vi "01 Washer HCC.vi"() -> ()   [LabVIEW 2009]
uses:
  Washer.ctl
  Dryer Wilt/Dryer Details.ctl
  Dryer Wilt/Dryer.ctl
  Dryer Wilt/Agilent Channel Definition.ctl
  Dryer Wilt/Dryer Com Port Info.ctl
  Dryer Wilt/Dryer Status Ctrl.ctl
  Dryer Wilt/Dryer Test State.ctl
  <vilib>/Platform/fileVersionInfo.llb/FileVersionInformation.ctl
  Globals HCC.vi
  Dryer Wilt/Update Wilt GUI Control.ctl
  Dryer Wilt/GEA2 Driver/GEA2 Dryer Interface Ctrl.ctl
panel:
  out "User Message":string
  in  "Reset Faults":bool
  in  "Save Setup":bool
  out "Agilent":T1
  out "File Version Info":string
  in  "Robocopy":bool
  out "4":T1
  out "3":T1
  out "2":T1
  out "1A":T1
  out "1":T1
  out "GUI Update":bool=TRUE
  out "Gathering Data Latch":bool=TRUE
  out "Init Complete":bool=TRUE
  out "Dryer Com Info":T2[](array[typedef])=[{"Color"=0, "Last Read Status"=enum."Cycle Not Started", "Command:Data"="", "Com Port"=0, "Time(S)"=0.0, "Err Count"=0}, {"Color"=0, "Last Read Status"=enum."Cycle Not Started", "Command:Data"="", "Com Port"=0, "Time(S)"=0.0, "Err Count"=0}, {"Color"=0, "Last Read Status"=enum."Cycle Not Started", "Command:Data"="", "Com Port"=0, "Time(S)"=0.0, "Err Count"=0}, {"Color"=0, "Last Read Status"=enum."Cycle Not Started", "Command:Data"="", "Com Port"=0, "Time(S)"=0.0, "Err Count"=0}, {"Color"=0, "Last Read Status"=enum."Cycle Not Started", "Command:Data"="", "Com Port"=0, "Time(S)"=0.0, "Err Count"=0}, {"Color"=0, "Last Read Status"=enum."Cycle Not Started", "Command:Data"="", "Com Port"=0, "Time(S)"=0.0, "Err Count"=0}, {"Color"=0, "Last Read Status"=enum."Cycle Not Started", "Command:Data"="", "Com Port"=0, "Time(S)"=0.0, "Err Count"=0}, {"Color"=0, "Last Read Status"=enum."Cycle Not Started", "Command:Data"="", "Com Port"=0, "Time(S)"=0.0, "Err Count"=0}, {"Color"=0, "Last Read Status"=enum."Cycle Not Started", "Command:Data"="", "Com Port"=0, "Time(S)"=0.0, "Err Count"=0}, {"Color"=0, "Last Read Status"=enum."Cycle Not Started", "Command:Data"="", "Com Port"=0, "Time(S)"=0.0, "Err Count"=0}, {"Color"=0, "Last Read Status"=enum."Cycle Not Started", "Command:Data"="", "Com Port"=0, "Time(S)"=0.0, "Err Count"=0}, {"Color"=0, "Last Read Status"=enum."Cycle Not Started", "Command:Data"="", "Com Port"=0, "Time(S)"=0.0, "Err Count"=0}, {"Color"=0, "Last Read Status"=enum."Cycle Not Started", "Command:Data"="", "Com Port"=0, "Time(S)"=0.0, "Err Count"=0}, {"Color"=0, "Last Read Status"=enum."Cycle Not Started", "Command:Data"="", "Com Port"=0, "Time(S)"=0.0, "Err Count"=0}, {"Color"=0, "Last Read Status"=enum."Cycle Not Started", "Command:Data"="", "Com Port"=0, "Time(S)"=0.0, "Err Count"=0}, {"Color"=0, "Last Read Status"=enum."Cycle Not Started", "Command:Data"="", "Com Port"=0, "Time(S)"=0.0, "Err Count"=0}, {"Color"=0, "Last Read Status"=enum."Cycle Not Started", "Command:Data"="", "Com Port"=0, "Time(S)"=0.0, "Err Count"=0}, {"Color"=0, "Last Read Status"=enum."Cycle Not Started", "Command:Data"="", "Com Port"=0, "Time(S)"=0.0, "Err Count"=0}, {"Color"=0, "Last Read Status"=enum."Cycle Not Started", "Command:Data"="", "Com Port"=0, "Time(S)"=0.0, "Err Count"=0}, {"Color"=0, "Last Read Status"=enum."Cycle Not Started", "Command:Data"="", "Com Port"=0, "Time(S)"=0.0, "Err Count"=0}, {"Color"=0, "Last Read Status"=enum."Cycle Not Started", "Command:Data"="", "Com Port"=0, "Time(S)"=0.0, "Err Count"=0}, {"Color"=0, "Last Read Status"=enum."Cycle Not Started", "Command:Data"="", "Com Port"=0, "Time(S)"=0.0, "Err Count"=0}, {"Color"=0, "Last Read Status"=enum."Cycle Not Started", "Command:Data"="", "Com Port"=0, "Time(S)"=0.0, "Err Count"=0}, {"Color"=0, "Last Read Status"=enum."Cycle Not Started", "Command:Data"="", "Com Port"=0, "Time(S)"=0.0, "Err Count"=0}, {"Color"=0, "Last Read Status"=enum."Cycle Not Started", "Command:Data"="", "Com Port"=0, "Time(S)"=0.0, "Err Count"=0}, {"Color"=0, "Last Read Status"=enum."Cycle Not Started", "Command:Data"="", "Com Port"=0, "Time(S)"=0.0, "Err Count"=0}, {"Color"=0, "Last Read Status"=enum."Cycle Not Started", "Command:Data"="", "Com Port"=0, "Time(S)"=0.0, "Err Count"=0}, {"Color"=0, "Last Read Status"=enum."Cycle Not Started", "Command:Data"="", "Com Port"=0, "Time(S)"=0.0, "Err Count"=0}, {"Color"=0, "Last Read Status"=enum."Cycle Not Started", "Command:Data"="", "Com Port"=0, "Time(S)"=0.0, "Err Count"=0}, {"Color"=0, "Last Read Status"=enum."Cycle Not Started", "Command:Data"="", "Com Port"=0, "Time(S)"=0.0, "Err Count"=0}, {"Color"=0, "Last Read Status"=enum."Cycle Not Started", "Command:Data"="", "Com Port"=0, "Time(S)"=0.0, "Err Count"=0}, {"Color"=0, "Last Read Status"=enum."Cycle Not Started", "Command:Data"="", "Com Port"=0, "Time(S)"=0.0, "Err Count"=0}, {"Color"=0, "Last Read Status"=enum."Cycle Not Started", "Command:Data"="", "Com Port"=0, "Time(S)"=0.0, "Err Count"=0}, {"Color"=0, "Last Read Status"=enum."Cycle Not Started", "Command:Data"="", "Com Port"=0, "Time(S)"=0.0, "Err Count"=0}, {"Color"=0, "Last Read Status"=enum."Cycle Not Started", "Command:Data"="", "Com Port"=0, "Time(S)"=0.0, "Err Count"=0}, {"Color"=0, "Last Read Status"=enum."Cycle Not Started", "Command:Data"="", "Com Port"=0, "Time(S)"=0.0, "Err Count"=0}, {"Color"=0, "Last Read Status"=enum."Cycle Not Started", "Command:Data"="", "Com Port"=0, "Time(S)"=0.0, "Err Count"=0}, {"Color"=0, "Last Read Status"=enum."Cycle Not Started", "Command:Data"="", "Com Port"=0, "Time(S)"=0.0, "Err Count"=0}, {"Color"=0, "Last Read Status"=enum."Cycle Not Started", "Command:Data"="", "Com Port"=0, "Time(S)"=0.0, "Err Count"=0}, {"Color"=0, "Last Read Status"=enum."Cycle Not Started", "Command:Data"="", "Com Port"=0, "Time(S)"=0.0, "Err Count"=0}, {"Color"=0, "Last Read Status"=enum."Cycle Not Started", "Command:Data"="", "Com Port"=0, "Time(S)"=0.0, "Err Count"=0}, {"Color"=0, "Last Read Status"=enum."Cycle Not Started", "Command:Data"="", "Com Port"=0, "Time(S)"=0.0, "Err Count"=0}, {"Color"=0, "Last Read Status"=enum."Cycle Not Started", "Command:Data"="", "Com Port"=0, "Time(S)"=0.0, "Err Count"=0}, {"Color"=0, "Last Read Status"=enum."Cycle Not Started", "Command:Data"="", "Com Port"=0, "Time(S)"=0.0, "Err Count"=0}, {"Color"=0, "Last Read Status"=enum."Cycle Not Started", "Command:Data"="", "Com Port"=0, "Time(S)"=0.0, "Err Count"=0}, {"Color"=0, "Last Read Status"=enum."Cycle Not Started", "Command:Data"="", "Com Port"=0, "Time(S)"=0.0, "Err Count"=0}, {"Color"=0, "Last Read Status"=enum."Cycle Not Started", "Command:Data"="", "Com Port"=0, "Time(S)"=0.0, "Err Count"=0}, {"Color"=0, "Last Read Status"=enum."Cycle Not Started", "Command:Data"="", "Com Port"=0, "Time(S)"=0.0, "Err Count"=0}, {"Color"=0, "Last Read Status"=enum."Cycle Not Started", "Command:Data"="", "Com Port"=0, "Time(S)"=0.0, "Err Count"=0}, {"Color"=0, "Last Read Status"=enum."Cycle Not Started", "Command:Data"="", "Com Port"=0, "Time(S)"=0.0, "Err Count"=0}, {"Color"=0, "Last Read Status"=enum."Cycle Not Started", "Command:Data"="", "Com Port"=0, "Time(S)"=0.0, "Err Count"=0}, {"Color"=0, "Last Read Status"=enum."Cycle Not Started", "Command:Data"="", "Com Port"=0, "Time(S)"=0.0, "Err Count"=0}, {"Color"=0, "Last Read Status"=enum."Cycle Not Started", "Command:Data"="", "Com Port"=0, "Time(S)"=0.0, "Err Count"=0}, {"Color"=0, "Last Read Status"=enum."Cycle Not Started", "Command:Data"="", "Com Port"=0, "Time(S)"=0.0, "Err Count"=0}, {"Color"=0, "Last Read Status"=enum."Cycle Not Started", "Command:Data"="", "Com Port"=0, "Time(S)"=0.0, "Err Count"=0}, {"Color"=0, "Last Read Status"=enum."Cycle Not Started", "Command:Data"="", "Com Port"=0, "Time(S)"=0.0, "Err Count"=0}, {"Color"=0, "Last Read Status"=enum."Cycle Not Started", "Command:Data"="", "Com Port"=0, "Time(S)"=0.0, "Err Count"=0}, {"Color"=0, "Last Read Status"=enum."Cycle Not Started", "Command:Data"="", "Com Port"=0, "Time(S)"=0.0, "Err Count"=0}, {"Color"=0, "Last Read Status"=enum."Cycle Not Started", "Command:Data"="", "Com Port"=0, "Time(S)"=0.0, "Err Count"=0}, {"Color"=0, "Last Read Status"=enum."Cycle Not Started", "Command:Data"="", "Com Port"=0, "Time(S)"=0.0, "Err Count"=0}, {"Color"=0, "Last Read Status"=enum."Cycle Not Started", "Command:Data"="", "Com Port"=0, "Time(S)"=0.0, "Err Count"=0}, {"Color"=0, "Last Read Status"=enum."Cycle Not Started", "Command:Data"="", "Com Port"=0, "Time(S)"=0.0, "Err Count"=0}, {"Color"=0, "Last Read Status"=enum."Cycle Not Started", "Command:Data"="", "Com Port"=0, "Time(S)"=0.0, "Err Count"=0}, {"Color"=0, "Last Read Status"=enum."Cycle Not Started", "Command:Data"="", "Com Port"=0, "Time(S)"=0.0, "Err Count"=0}, {"Color"=0, "Last Read Status"=enum."Cycle Not Started", "Command:Data"="", "Com Port"=0, "Time(S)"=0.0, "Err Count"=0}, {"Color"=0, "Last Read Status"=enum."Cycle Not Started", "Command:Data"="", "Com Port"=0, "Time(S)"=0.0, "Err Count"=0}, {"Color"=0, "Last Read Status"=enum."Cycle Not Started", "Command:Data"="", "Com Port"=0, "Time(S)"=0.0, "Err Count"=0}, {"Color"=0, "Last Read Status"=enum."Cycle Not Started", "Command:Data"="", "Com Port"=0, "Time(S)"=0.0, "Err Count"=0}, {"Color"=0, "Last Read Status"=enum."Cycle Not Started", "Command:Data"="", "Com Port"=0, "Time(S)"=0.0, "Err Count"=0}, {"Color"=0, "Last Read Status"=enum."Cycle Not Started", "Command:Data"="", "Com Port"=0, "Time(S)"=0.0, "Err Count"=0}, {"Color"=0, "Last Read Status"=enum."Cycle Not Started", "Command:Data"="", "Com Port"=0, "Time(S)"=0.0, "Err Count"=0}, {"Color"=0, "Last Read Status"=enum."Cycle Not Started", "Command:Data"="", "Com Port"=0, "Time(S)"=0.0, "Err Count"=0}, {"Color"=0, "Last Read Status"=enum."Cycle Not Started", "Command:Data"="", "Com Port"=0, "Time(S)"=0.0, "Err Count"=0}, {"Color"=0, "Last Read Status"=enum."Cycle Not Started", "Command:Data"="", "Com Port"=0, "Time(S)"=0.0, "Err Count"=0}, {"Color"=0, "Last Read Status"=enum."Cycle Not Started", "Command:Data"="", "Com Port"=0, "Time(S)"=0.0, "Err Count"=0}, {"Color"=0, "Last Read Status"=enum."Cycle Not Started", "Command:Data"="", "Com Port"=0, "Time(S)"=0.0, "Err Count"=0}, {"Color"=0, "Last Read Status"=enum."Cycle Not Started", "Command:Data"="", "Com Port"=0, "Time(S)"=0.0, "Err Count"=0}, {"Color"=0, "Last Read Status"=enum."Cycle Not Started", "Command:Data"="", "Com Port"=0, "Time(S)"=0.0, "Err Count"=0}, {"Color"=0, "Last Read Status"=enum."Cycle Not Started", "Command:Data"="", "Com Port"=0, "Time(S)"=0.0, "Err Count"=0}, {"Color"=0, "Last Read Status"=enum."Cycle Not Started", "Command:Data"="", "Com Port"=0, "Time(S)"=0.0, "Err Count"=0}, {"Color"=0, "Last Read Status"=enum."Cycle Not Started", "Command:Data"="", "Com Port"=0, "Time(S)"=0.0, "Err Count"=0}, {"Color"=0, "Last Read Status"=enum."Cycle Not Started", "Command:Data"="", "Com Port"=0, "Time(S)"=0.0, "Err Count"=0}, {"Color"=0, "Last Read Status"=enum."Cycle Not Started", "Command:Data"="", "Com Port"=0, "Time(S)"=0.0, "Err Count"=0}, {"Color"=0, "Last Read Status"=enum."Cycle Not Started", "Command:Data"="", "Com Port"=0, "Time(S)"=0.0, "Err Count"=0}, {"Color"=0, "Last Read Status"=enum."Cycle Not Started", "Command:Data"="", "Com Port"=0, "Time(S)"=0.0, "Err Count"=0}, {"Color"=0, "Last Read Status"=enum."Cycle Not Started", "Command:Data"="", "Com Port"=0, "Time(S)"=0.0, "Err Count"=0}, {"Color"=0, "Last Read Status"=enum."Cycle Not Started", "Command:Data"="", "Com Port"=0, "Time(S)"=0.0, "Err Count"=0}, {"Color"=0, "Last Read Status"=enum."Cycle Not Started", "Command:Data"="", "Com Port"=0, "Time(S)"=0.0, "Err Count"=0}, {"Color"=0, "Last Read Status"=enum."Cycle Not Started", "Command:Data"="", "Com Port"=0, "Time(S)"=0.0, "Err Count"=0}, {"Color"=0, "Last Read Status"=enum."Cycle Not Started", "Command:Data"="", "Com Port"=0, "Time(S)"=0.0, "Err Count"=0}, {"Color"=0, "Last Read Status"=enum."Cycle Not Started", "Command:Data"="", "Com Port"=0, "Time(S)"=0.0, "Err Count"=0}, {"Color"=0, "Last Read Status"=enum."Cycle Not Started", "Command:Data"="", "Com Port"=0, "Time(S)"=0.0, "Err Count"=0}, {"Color"=0, "Last Read Status"=enum."Cycle Not Started", "Command:Data"="", "Com Port"=0, "Time(S)"=0.0, "Err Count"=0}, {"Color"=0, "Last Read Status"=enum."Cycle Not Started", "Command:Data"="", "Com Port"=0, "Time(S)"=0.0, "Err Count"=0}, {"Color"=0, "Last Read Status"=enum."Cycle Not Started", "Command:Data"="", "Com Port"=0, "Time(S)"=0.0, "Err Count"=0}, {"Color"=0, "Last Read Status"=enum."Cycle Not Started", "Command:Data"="", "Com Port"=0, "Time(S)"=0.0, "Err Count"=0}, {"Color"=0, "Last Read Status"=enum."Cycle Not Started", "Command:Data"="", "Com Port"=0, "Time(S)"=0.0, "Err Count"=0}, {"Color"=0, "Last Read Status"=enum."Cycle Not Started", "Command:Data"="", "Com Port"=0, "Time(S)"=0.0, "Err Count"=0}, {"Color"=0, "Last Read Status"=enum."Cycle Not Started", "Command:Data"="", "Com Port"=0, "Time(S)"=0.0, "Err Count"=0}, {"Color"=0, "Last Read Status"=enum."Cycle Not Started", "Command:Data"="", "Com Port"=0, "Time(S)"=0.0, "Err Count"=0}, {"Color"=0, "Last Read Status"=enum."Cycle Not Started", "Command:Data"="", "Com Port"=0, "Time(S)"=0.0, "Err Count"=0}, {"Color"=0, "Last Read Status"=enum."Cycle Not Started", "Command:Data"="", "Com Port"=0, "Time(S)"=0.0, "Err Count"=0}, {"Color"=0, "Last Read Status"=enum."Cycle Not Started", "Command:Data"="", "Com Port"=0, "Time(S)"=0.0, "Err Count"=0}, {"Color"=0, "Last Read Status"=enum."Cycle Not Started", "Command:Data"="", "Com Port"=0, "Time(S)"=0.0, "Err Count"=0}, {"Color"=0, "Last Read Status"=enum."Cycle Not Started", "Command:Data"="", "Com Port"=0, "Time(S)"=0.0, "Err Count"=0}, {"Color"=0, "Last Read Status"=enum."Cycle Not Started", "Command:Data"="", "Com Port"=0, "Time(S)"=0.0, "Err Count"=0}, {"Color"=0, "Last Read Status"=enum."Cycle Not Started", "Command:Data"="", "Com Port"=0, "Time(S)"=0.0, "Err Count"=0}, {"Color"=0, "Last Read Status"=enum."Cycle Not Started", "Command:Data"="", "Com Port"=0, "Time(S)"=0.0, "Err Count"=0}, {"Color"=0, "Last Read Status"=enum."Cycle Not Started", "Command:Data"="", "Com Port"=0, "Time(S)"=0.0, "Err Count"=0}, {"Color"=0, "Last Read Status"=enum."Cycle Not Started", "Command:Data"="", "Com Port"=0, "Time(S)"=0.0, "Err Count"=0}, {"Color"=0, "Last Read Status"=enum."Cycle Not Started", "Command:Data"="", "Com Port"=0, "Time(S)"=0.0, "Err Count"=0}, {"Color"=0, "Last Read Status"=enum."Cycle Not Started", "Command:Data"="", "Com Port"=0, "Time(S)"=0.0, "Err Count"=0}, {"Color"=0, "Last Read Status"=enum."Cycle Not Started", "Command:Data"="", "Com Port"=0, "Time(S)"=0.0, "Err Count"=0}, {"Color"=0, "Last Read Status"=enum."Cycle Not Started", "Command:Data"="", "Com Port"=0, "Time(S)"=0.0, "Err Count"=0}, {"Color"=0, "Last Read Status"=enum."Cycle Not Started", "Command:Data"="", "Com Port"=0, "Time(S)"=0.0, "Err Count"=0}, {"Color"=0, "Last Read Status"=enum."Cycle Not Started", "Command:Data"="", "Com Port"=0, "Time(S)"=0.0, "Err Count"=0}, {"Color"=0, "Last Read Status"=enum."Cycle Not Started", "Command:Data"="", "Com Port"=0, "Time(S)"=0.0, "Err Count"=0}, {"Color"=0, "Last Read Status"=enum."Cycle Not Started", "Command:Data"="", "Com Port"=0, "Time(S)"=0.0, "Err Count"=0}, {"Color"=0, "Last Read Status"=enum."Cycle Not Started", "Command:Data"="", "Com Port"=0, "Time(S)"=0.0, "Err Count"=0}, {"Color"=0, "Last Read Status"=enum."Cycle Not Started", "Command:Data"="", "Com Port"=0, "Time(S)"=0.0, "Err Count"=0}, {"Color"=0, "Last Read Status"=enum."Cycle Not Started", "Command:Data"="", "Com Port"=0, "Time(S)"=0.0, "Err Count"=0}, {"Color"=0, "Last Read Status"=enum."Cycle Not Started", "Command:Data"="", "Com Port"=0, "Time(S)"=0.0, "Err Count"=0}, {"Color"=0, "Last Read Status"=enum."Cycle Not Started", "Command:Data"="", "Com Port"=0, "Time(S)"=0.0, "Err Count"=0}, {"Color"=0, "Last Read Status"=enum."Cycle Not Started", "Command:Data"="", "Com Port"=0, "Time(S)"=0.0, "Err Count"=0}, {"Color"=0, "Last Read Status"=enum."Cycle Not Started", "Command:Data"="", "Com Port"=0, "Time(S)"=0.0, "Err Count"=0}, {"Color"=0, "Last Read Status"=enum."Cycle Not Started", "Command:Data"="", "Com Port"=0, "Time(S)"=0.0, "Err Count"=0}, {"Color"=0, "Last Read Status"=enum."Cycle Not Started", "Command:Data"="", "Com Port"=0, "Time(S)"=0.0, "Err Count"=0}, {"Color"=0, "Last Read Status"=enum."Cycle Not Started", "Command:Data"="", "Com Port"=0, "Time(S)"=0.0, "Err Count"=0}, {"Color"=0, "Last Read Status"=enum."Cycle Not Started", "Command:Data"="", "Com Port"=0, "Time(S)"=0.0, "Err Count"=0}, {"Color"=0, "Last Read Status"=enum."Cycle Not Started", "Command:Data"="", "Com Port"=0, "Time(S)"=0.0, "Err Count"=0}, {"Color"=0, "Last Read Status"=enum."Cycle Not Started", "Command:Data"="", "Com Port"=0, "Time(S)"=0.0, "Err Count"=0}, {"Color"=0, "Last Read Status"=enum."Cycle Not Started", "Command:Data"="", "Com Port"=0, "Time(S)"=0.0, "Err Count"=0}, {"Color"=0, "Last Read Status"=enum."Cycle Not Started", "Command:Data"="", "Com Port"=0, "Time(S)"=0.0, "Err Count"=0}, {"Color"=0, "Last Read Status"=enum."Cycle Not Started", "Command:Data"="", "Com Port"=0, "Time(S)"=0.0, "Err Count"=0}, {"Color"=0, "Last Read Status"=enum."Cycle Not Started", "Command:Data"="", "Com Port"=0, "Time(S)"=0.0, "Err Count"=0}, {"Color"=0, "Last Read Status"=enum."Cycle Not Started", "Command:Data"="", "Com Port"=0, "Time(S)"=0.0, "Err Count"=0}, {"Color"=0, "Last Read Status"=enum."Cycle Not Started", "Command:Data"="", "Com Port"=0, "Time(S)"=0.0, "Err Count"=0}, {"Color"=0, "Last Read Status"=enum."Cycle Not Started", "Command:Data"="", "Com Port"=0, "Time(S)"=0.0, "Err Count"=0}, {"Color"=0, "Last Read Status"=enum."Cycle Not Started", "Command:Data"="", "Com Port"=0, "Time(S)"=0.0, "Err Count"=0}, {"Color"=0, "Last Read Status"=enum."Cycle Not Started", "Command:Data"="", "Com Port"=0, "Time(S)"=0.0, "Err Count"=0}, {"Color"=0, "Last Read Status"=enum."Cycle Not Started", "Command:Data"="", "Com Port"=0, "Time(S)"=0.0, "Err Count"=0}, {"Color"=0, "Last Read Status"=enum."Cycle Not Started", "Command:Data"="", "Com Port"=0, "Time(S)"=0.0, "Err Count"=0}, {"Color"=0, "Last Read Status"=enum."Cycle Not Started", "Command:Data"="", "Com Port"=0, "Time(S)"=0.0, "Err Count"=0}, {"Color"=0, "Last Read Status"=enum."Cycle Not Started", "Command:Data"="", "Com Port"=0, "Time(S)"=0.0, "Err Count"=0}, {"Color"=0, "Last Read Status"=enum."Cycle Not Started", "Command:Data"="", "Com Port"=0, "Time(S)"=0.0, "Err Count"=0}, {"Color"=0, "Last Read Status"=enum."Cycle Not Started", "Command:Data"="", "Com Port"=0, "Time(S)"=0.0, "Err Count"=0}, {"Color"=0, "Last Read Status"=enum."Cycle Not Started", "Command:Data"="", "Com Port"=0, "Time(S)"=0.0, "Err Count"=0}, {"Color"=0, "Last Read Status"=enum."Cycle Not Started", "Command:Data"="", "Com Port"=0, "Time(S)"=0.0, "Err Count"=0}, {"Color"=0, "Last Read Status"=enum."Cycle Not Started", "Command:Data"="", "Com Port"=0, "Time(S)"=0.0, "Err Count"=0}, {"Color"=0, "Last Read Status"=enum."Cycle Not Started", "Command:Data"="", "Com Port"=0, "Time(S)"=0.0, "Err Count"=0}, {"Color"=0, "Last Read Status"=enum."Cycle Not Started", "Command:Data"="", "Com Port"=0, "Time(S)"=0.0, "Err Count"=0}, {"Color"=0, "Last Read Status"=enum."Cycle Not Started", "Command:Data"="", "Com Port"=0, "Time(S)"=0.0, "Err Count"=0}, {"Color"=0, "Last Read Status"=enum."Cycle Not Started", "Command:Data"="", "Com Port"=0, "Time(S)"=0.0, "Err Count"=0}, {"Color"=0, "Last Read Status"=enum."Cycle Not Started", "Command:Data"="", "Com Port"=0, "Time(S)"=0.0, "Err Count"=0}, {"Color"=0, "Last Read Status"=enum."Cycle Not Started", "Command:Data"="", "Com Port"=0, "Time(S)"=0.0, "Err Count"=0}, {"Color"=0, "Last Read Status"=enum."Cycle Not Started", "Command:Data"="", "Com Port"=0, "Time(S)"=0.0, "Err Count"=0}, {"Color"=0, "Last Read Status"=enum."Cycle Not Started", "Command:Data"="", "Com Port"=0, "Time(S)"=0.0, "Err Count"=0}, {"Color"=0, "Last Read Status"=enum."Cycle Not Started", "Command:Data"="", "Com Port"=0, "Time(S)"=0.0, "Err Count"=0}, {"Color"=0, "Last Read Status"=enum."Cycle Not Started", "Command:Data"="", "Com Port"=0, "Time(S)"=0.0, "Err Count"=0}, {"Color"=0, "Last Read Status"=enum."Cycle Not Started", "Command:Data"="", "Com Port"=0, "Time(S)"=0.0, "Err Count"=0}, {"Color"=0, "Last Read Status"=enum."Cycle Not Started", "Command:Data"="", "Com Port"=0, "Time(S)"=0.0, "Err Count"=0}, {"Color"=0, "Last Read Status"=enum."Cycle Not Started", "Command:Data"="", "Com Port"=0, "Time(S)"=0.0, "Err Count"=0}, {"Color"=0, "Last Read Status"=enum."Cycle Not Started", "Command:Data"="", "Com Port"=0, "Time(S)"=0.0, "Err Count"=0}, {"Color"=0, "Last Read Status"=enum."Cycle Not Started", "Command:Data"="", "Com Port"=0, "Time(S)"=0.0, "Err Count"=0}, {"Color"=0, "Last Read Status"=enum."Cycle Not Started", "Command:Data"="", "Com Port"=0, "Time(S)"=0.0, "Err Count"=0}, {"Color"=0, "Last Read Status"=enum."Cycle Not Started", "Command:Data"="", "Com Port"=0, "Time(S)"=0.0, "Err Count"=0}, {"Color"=0, "Last Read Status"=enum."Cycle Not Started", "Command:Data"="", "Com Port"=0, "Time(S)"=0.0, "Err Count"=0}, {"Color"=0, "Last Read Status"=enum."Cycle Not Started", "Command:Data"="", "Com Port"=0, "Time(S)"=0.0, "Err Count"=0}, {"Color"=0, "Last Read Status"=enum."Cycle Not Started", "Command:Data"="", "Com Port"=0, "Time(S)"=0.0, "Err Count"=0}, {"Color"=0, "Last Read Status"=enum."Cycle Not Started", "Command:Data"="", "Com Port"=0, "Time(S)"=0.0, "Err Count"=0}, {"Color"=0, "Last Read Status"=enum."Cycle Not Started", "Command:Data"="", "Com Port"=0, "Time(S)"=0.0, "Err Count"=0}, {"Color"=0, "Last Read Status"=enum."Cycle Not Started", "Command:Data"="", "Com Port"=0, "Time(S)"=0.0, "Err Count"=0}, {"Color"=0, "Last Read Status"=enum."Cycle Not Started", "Command:Data"="", "Com Port"=0, "Time(S)"=0.0, "Err Count"=0}, {"Color"=0, "Last Read Status"=enum."Cycle Not Started", "Command:Data"="", "Com Port"=0, "Time(S)"=0.0, "Err Count"=0}, {"Color"=0, "Last Read Status"=enum."Cycle Not Started", "Command:Data"="", "Com Port"=0, "Time(S)"=0.0, "Err Count"=0}, {"Color"=0, "Last Read Status"=enum."Cycle Not Started", "Command:Data"="", "Com Port"=0, "Time(S)"=0.0, "Err Count"=0}, {"Color"=0, "Last Read Status"=enum."Cycle Not Started", "Command:Data"="", "Com Port"=0, "Time(S)"=0.0, "Err Count"=0}, {"Color"=0, "Last Read Status"=enum."Cycle Not Started", "Command:Data"="", "Com Port"=0, "Time(S)"=0.0, "Err Count"=0}, {"Color"=0, "Last Read Status"=enum."Cycle Not Started", "Command:Data"="", "Com Port"=0, "Time(S)"=0.0, "Err Count"=0}, {"Color"=0, "Last Read Status"=enum."Cycle Not Started", "Command:Data"="", "Com Port"=0, "Time(S)"=0.0, "Err Count"=0}, {"Color"=0, "Last Read Status"=enum."Cycle Not Started", "Command:Data"="", "Com Port"=0, "Time(S)"=0.0, "Err Count"=0}, {"Color"=0, "Last Read Status"=enum."Cycle Not Started", "Command:Data"="", "Com Port"=0, "Time(S)"=0.0, "Err Count"=0}, {"Color"=0, "Last Read Status"=enum."Cycle Not Started", "Command:Data"="", "Com Port"=0, "Time(S)"=0.0, "Err Count"=0}, {"Color"=0, "Last Read Status"=enum."Cycle Not Started", "Command:Data"="", "Com Port"=0, "Time(S)"=0.0, "Err Count"=0}, {"Color"=0, "Last Read Status"=enum."Cycle Not Started", "Command:Data"="", "Com Port"=0, "Time(S)"=0.0, "Err Count"=0}, {"Color"=0, "Last Read Status"=enum."Cycle Not Started", "Command:Data"="", "Com Port"=0, "Time(S)"=0.0, "Err Count"=0}, {"Color"=0, "Last Read Status"=enum."Cycle Not Started", "Command:Data"="", "Com Port"=0, "Time(S)"=0.0, "Err Count"=0}, {"Color"=0, "Last Read Status"=enum."Cycle Not Started", "Command:Data"="", "Com Port"=0, "Time(S)"=0.0, "Err Count"=0}, {"Color"=0, "Last Read Status"=enum."Cycle Not Started", "Command:Data"="", "Com Port"=0, "Time(S)"=0.0, "Err Count"=0}, {"Color"=0, "Last Read Status"=enum."Cycle Not Started", "Command:Data"="", "Com Port"=0, "Time(S)"=0.0, "Err Count"=0}, {"Color"=0, "Last Read Status"=enum."Cycle Not Started", "Command:Data"="", "Com Port"=0, "Time(S)"=0.0, "Err Count"=0}, {"Color"=0, "Last Read Status"=enum."Cycle Not Started", "Command:Data"="", "Com Port"=0, "Time(S)"=0.0, "Err Count"=0}, {"Color"=0, "Last Read Status"=enum."Cycle Not Started", "Command:Data"="", "Com Port"=0, "Time(S)"=0.0, "Err Count"=0}, {"Color"=0, "Last Read Status"=enum."Cycle Not Started", "Command:Data"="", "Com Port"=0, "Time(S)"=0.0, "Err Count"=0}, {"Color"=0, "Last Read Status"=enum."Cycle Not Started", "Command:Data"="", "Com Port"=0, "Time(S)"=0.0, "Err Count"=0}, {"Color"=0, "Last Read Status"=enum."Cycle Not Started", "Command:Data"="", "Com Port"=0, "Time(S)"=0.0, "Err Count"=0}, {"Color"=0, "Last Read Status"=enum."Cycle Not Started", "Command:Data"="", "Com Port"=0, "Time(S)"=0.0, "Err Count"=0}, {"Color"=0, "Last Read Status"=enum."Cycle Not Started", "Command:Data"="", "Com Port"=0, "Time(S)"=0.0, "Err Count"=0}, {"Color"=0, "Last Read Status"=enum."Cycle Not Started", "Command:Data"="", "Com Port"=0, "Time(S)"=0.0, "Err Count"=0}, {"Color"=0, "Last Read Status"=enum."Cycle Not Started", "Command:Data"="", "Com Port"=0, "Time(S)"=0.0, "Err Count"=0}, {"Color"=0, "Last Read Status"=enum."Cycle Not Started", "Command:Data"="", "Com Port"=0, "Time(S)"=0.0, "Err Count"=0}, {"Color"=0, "Last Read Status"=enum."Cycle Not Started", "Command:Data"="", "Com Port"=0, "Time(S)"=0.0, "Err Count"=0}, {"Color"=0, "Last Read Status"=enum."Cycle Not Started", "Command:Data"="", "Com Port"=0, "Time(S)"=0.0, "Err Count"=0}, {"Color"=0, "Last Read Status"=enum."Cycle Not Started", "Command:Data"="", "Com Port"=0, "Time(S)"=0.0, "Err Count"=0}, {"Color"=0, "Last Read Status"=enum."Cycle Not Started", "Command:Data"="", "Com Port"=0, "Time(S)"=0.0, "Err Count"=0}, {"Color"=0, "Last Read Status"=enum."Cycle Not Started", "Command:Data"="", "Com Port"=0, "Time(S)"=0.0, "Err Count"=0}, {"Color"=0, "Last Read Status"=enum."Cycle Not Started", "Command:Data"="", "Com Port"=0, "Time(S)"=0.0, "Err Count"=0}, {"Color"=0, "Last Read Status"=enum."Cycle Not Started", "Command:Data"="", "Com Port"=0, "Time(S)"=0.0, "Err Count"=0}, {"Color"=0, "Last Read Status"=enum."Cycle Not Started", "Command:Data"="", "Com Port"=0, "Time(S)"=0.0, "Err Count"=0}, {"Color"=0, "Last Read Status"=enum."Cycle Not Started", "Command:Data"="", "Com Port"=0, "Time(S)"=0.0, "Err Count"=0}, {"Color"=0, "Last Read Status"=enum."Cycle Not Started", "Command:Data"="", "Com Port"=0, "Time(S)"=0.0, "Err Count"=0}, {"Color"=0, "Last Read Status"=enum."Cycle Not Started", "Command:Data"="", "Com Port"=0, "Time(S)"=0.0, "Err Count"=0}, {"Color"=0, "Last Read Status"=enum."Cycle Not Started", "Command:Data"="", "Com Port"=0, "Time(S)"=0.0, "Err Count"=0}, {"Color"=0, "Last Read Status"=enum."Cycle Not Started", "Command:Data"="", "Com Port"=0, "Time(S)"=0.0, "Err Count"=0}, {"Color"=0, "Last Read Status"=enum."Cycle Not Started", "Command:Data"="", "Com Port"=0, "Time(S)"=0.0, "Err Count"=0}, {"Color"=0, "Last Read Status"=enum."Cycle Not Started", "Command:Data"="", "Com Port"=0, "Time(S)"=0.0, "Err Count"=0}, {"Color"=0, "Last Read Status"=enum."Cycle Not Started", "Command:Data"="", "Com Port"=0, "Time(S)"=0.0, "Err Count"=0}, {"Color"=0, "Last Read Status"=enum."Cycle Not Started", "Command:Data"="", "Com Port"=0, "Time(S)"=0.0, "Err Count"=0}, {"Color"=0, "Last Read Status"=enum."Cycle Not Started", "Command:Data"="", "Com Port"=0, "Time(S)"=0.0, "Err Count"=0}, {"Color"=0, "Last Read Status"=enum."Cycle Not Started", "Command:Data"="", "Com Port"=0, "Time(S)"=0.0, "Err Count"=0}, {"Color"=0, "Last Read Status"=enum."Cycle Not Started", "Command:Data"="", "Com Port"=0, "Time(S)"=0.0, "Err Count"=0}, {"Color"=0, "Last Read Status"=enum."Cycle Not Started", "Command:Data"="", "Com Port"=0, "Time(S)"=0.0, "Err Count"=0}, {"Color"=0, "Last Read Status"=enum."Cycle Not Started", "Command:Data"="", "Com Port"=0, "Time(S)"=0.0, "Err Count"=0}, {"Color"=0, "Last Read Status"=enum."Cycle Not Started", "Command:Data"="", "Com Port"=0, "Time(S)"=0.0, "Err Count"=0}, {"Color"=0, "Last Read Status"=enum."Cycle Not Started", "Command:Data"="", "Com Port"=0, "Time(S)"=0.0, "Err Count"=0}, {"Color"=0, "Last Read Status"=enum."Cycle Not Started", "Command:Data"="", "Com Port"=0, "Time(S)"=0.0, "Err Count"=0}, {"Color"=0, "Last Read Status"=enum."Cycle Not Started", "Command:Data"="", "Com Port"=0, "Time(S)"=0.0, "Err Count"=0}, {"Color"=0, "Last Read Status"=enum."Cycle Not Started", "Command:Data"="", "Com Port"=0, "Time(S)"=0.0, "Err Count"=0}, {"Color"=0, "Last Read Status"=enum."Cycle Not Started", "Command:Data"="", "Com Port"=0, "Time(S)"=0.0, "Err Count"=0}, {"Color"=0, "Last Read Status"=enum."Cycle Not Started", "Command:Data"="", "Com Port"=0, "Time(S)"=0.0, "Err Count"=0}, {"Color"=0, "Last Read Status"=enum."Cycle Not Started", "Command:Data"="", "Com Port"=0, "Time(S)"=0.0, "Err Count"=0}, {"Color"=0, "Last Read Status"=enum."Cycle Not Started", "Command:Data"="", "Com Port"=0, "Time(S)"=0.0, "Err Count"=0}, {"Color"=0, "Last Read Status"=enum."Cycle Not Started", "Command:Data"="", "Com Port"=0, "Time(S)"=0.0, "Err Count"=0}, {"Color"=0, "Last Read Status"=enum."Cycle Not Started", "Command:Data"="", "Com Port"=0, "Time(S)"=0.0, "Err Count"=0}, {"Color"=0, "Last Read Status"=enum."Cycle Not Started", "Command:Data"="", "Com Port"=0, "Time(S)"=0.0, "Err Count"=0}, {"Color"=0, "Last Read Status"=enum."Cycle Not Started", "Command:Data"="", "Com Port"=0, "Time(S)"=0.0, "Err Count"=0}, {"Color"=0, "Last Read Status"=enum."Cycle Not Started", "Command:Data"="", "Com Port"=0, "Time(S)"=0.0, "Err Count"=0}, {"Color"=0, "Last Read Status"=enum."Cycle Not Started", "Command:Data"="", "Com Port"=0, "Time(S)"=0.0, "Err Count"=0}, {"Color"=0, "Last Read Status"=enum."Cycle Not Started", "Command:Data"="", "Com Port"=0, "Time(S)"=0.0, "Err Count"=0}, {"Color"=0, "Last Read Status"=enum."Cycle Not Started", "Command:Data"="", "Com Port"=0, "Time(S)"=0.0, "Err Count"=0}, {"Color"=0, "Last Read Status"=enum."Cycle Not Started", "Command:Data"="", "Com Port"=0, "Time(S)"=0.0, "Err Count"=0}, {"Color"=0, "Last Read Status"=enum."Cycle Not Started", "Command:Data"="", "Com Port"=0, "Time(S)"=0.0, "Err Count"=0}, {"Color"=0, "Last Read Status"=enum."Cycle Not Started", "Command:Data"="", "Com Port"=0, "Time(S)"=0.0, "Err Count"=0}, {"Color"=0, "Last Read Status"=enum."Cycle Not Started", "Command:Data"="", "Com Port"=0, "Time(S)"=0.0, "Err Count"=0}, {"Color"=0, "Last Read Status"=enum."Cycle Not Started", "Command:Data"="", "Com Port"=0, "Time(S)"=0.0, "Err Count"=0}, {"Color"=0, "Last Read Status"=enum."Cycle Not Started", "Command:Data"="", "Com Port"=0, "Time(S)"=0.0, "Err Count"=0}, {"Color"=0, "Last Read Status"=enum."Cycle Not Started", "Command:Data"="", "Com Port"=0, "Time(S)"=0.0, "Err Count"=0}, {"Color"=0, "Last Read Status"=enum."Cycle Not Started", "Command:Data"="", "Com Port"=0, "Time(S)"=0.0, "Err Count"=0}, {"Color"=0, "Last Read Status"=enum."Cycle Not Started", "Command:Data"="", "Com Port"=0, "Time(S)"=0.0, "Err Count"=0}, {"Color"=0, "Last Read Status"=enum."Cycle Not Started", "Command:Data"="", "Com Port"=0, "Time(S)"=0.0, "Err Count"=0}, {"Color"=0, "Last Read Status"=enum."Cycle Not Started", "Command:Data"="", "Com Port"=0, "Time(S)"=0.0, "Err Count"=0}, {"Color"=0, "Last Read Status"=enum."Cycle Not Started", "Command:Data"="", "Com Port"=0, "Time(S)"=0.0, "Err Count"=0}, {"Color"=0, "Last Read Status"=enum."Cycle Not Started", "Command:Data"="", "Com Port"=0, "Time(S)"=0.0, "Err Count"=0}, {"Color"=0, "Last Read Status"=enum."Cycle Not Started", "Command:Data"="", "Com Port"=0, "Time(S)"=0.0, "Err Count"=0}, {"Color"=0, "Last Read Status"=enum."Cycle Not Started", "Command:Data"="", "Com Port"=0, "Time(S)"=0.0, "Err Count"=0}, {"Color"=0, "Last Read Status"=enum."Cycle Not Started", "Command:Data"="", "Com Port"=0, "Time(S)"=0.0, "Err Count"=0}, {"Color"=0, "Last Read Status"=enum."Cycle Not Started", "Command:Data"="", "Com Port"=0, "Time(S)"=0.0, "Err Count"=0}]
  in  "GUI Aisle Bot":T4[](array[typedef]) {"Cycle Count" format="%05d"}
  in  "GUI Aisle Mid":T4[](array[typedef]) {"Cycle Count" format="%05d"}
  in  "GUI Aisle Top":T4[](array[typedef]) {"Cycle Count" format="%05d"}
  out "Elapsed Time (sec)":dbl format="%<%H:%M:%S>t"
  in  "Tab Control":T6(tab)=enum."Directories"
  in  "DAQ Delay":u32=1000
  out "All Confgured Com Array":u8[](array[numeric])=[100, 2, 3, 4, 5, 6, 7, 8, 9, 10, 11, 12, 13, 14, 15, 16, 17, 18, 19, 20, 21, 22, 23, 24, 25, 26, 27, 28, 29, 30, 31, 32, 33, 34, 35, 36, 37, 38, 39, 40, 41, 42, 43, 44, 45, 46, 47, 48, 49, 50, 51, 52, 53, 54, 55, 56]
  out "Test Complete":bool
  in  "Debug":bool
  in  "Dryer To Save":T7 {"Station Number" format="%02.0f"; "Cycle Count" format="%05d"}
  in  "Station Timer":dbl[](array[numeric])
  out "Log Coms Array":string[](array[string])
  in  "Data Sample File Directory":path=path "C:/data/Wilt Sample Data"
  in  "Dryer Bank Filename":path=path "C:/data/Wilt Backup"
  in  "Data Hist File Directory":path=path "C:/data/Wilt Hist/WiltHist.txt"
  in  "Data Sample File":path=path "C:/data/Wilt Sample Data"
  in  "Agilent Channel Assignment":path=path "C:/data/Agilent Channel Assignment - Wilt.ini"
  out "FileVersionInfo Out":T8
  in  "Station Com List":u8[](array[numeric])
  out "Current Agilent Data":dbl[](array[numeric])
  out "Agilent Station Data Index Array":i32[][](array[numeric])
  out "Agilent Read Channels Array":T9[](array[typedef])
  out "Agilent Station Data Headers":string[][](array[string])
  out "All Agilent Refs":refnum<visa-resource-name>[](array[refnum])=["AGILENT1", "AGILENT2", "AGILENT3", "AGILENT4", "AGILENT5"]
  out "Agilent Read Refs":refnum<visa-resource-name>[](array[refnum])=["AGILENT1", "AGILENT2", "AGILENT3", "AGILENT4", "AGILENT5"]
  out "Agilent Channels Water Valves":T9[](array[typedef])
  in  "Wait Com Timer":dbl=15.0
  out "All Test Stations":T4[](array[typedef]) {"Cycle Count" format="%05d"}
  out "Agilent Read Errors":errorcluster
  in  "Resend Start Limit":dbl=60.0
  in  "Saved Test State":T10[](array[typedef])
  in  "Station Test State":T10[](array[typedef])
  in  "Cooldown time":dbl=30.0
  out "GUI":string
  out "Daq":string
  out "Test State array":string[](array[string])
  out "Current State":string
  out "WC Bytes":u32
  out "WC x > 0?":bool
  out "DAQ Error List":string
  out "Control Error List":string
  out "UI Error List":string
  in  "Stop Test":bool
  out "Fault":u32(colorbox)=16711680
  out "Stopped":u32(colorbox)=16776960
  out "Running":u32(colorbox)=6618880
  out "No Com":u32(colorbox)
  # "HCC WASHER Test"
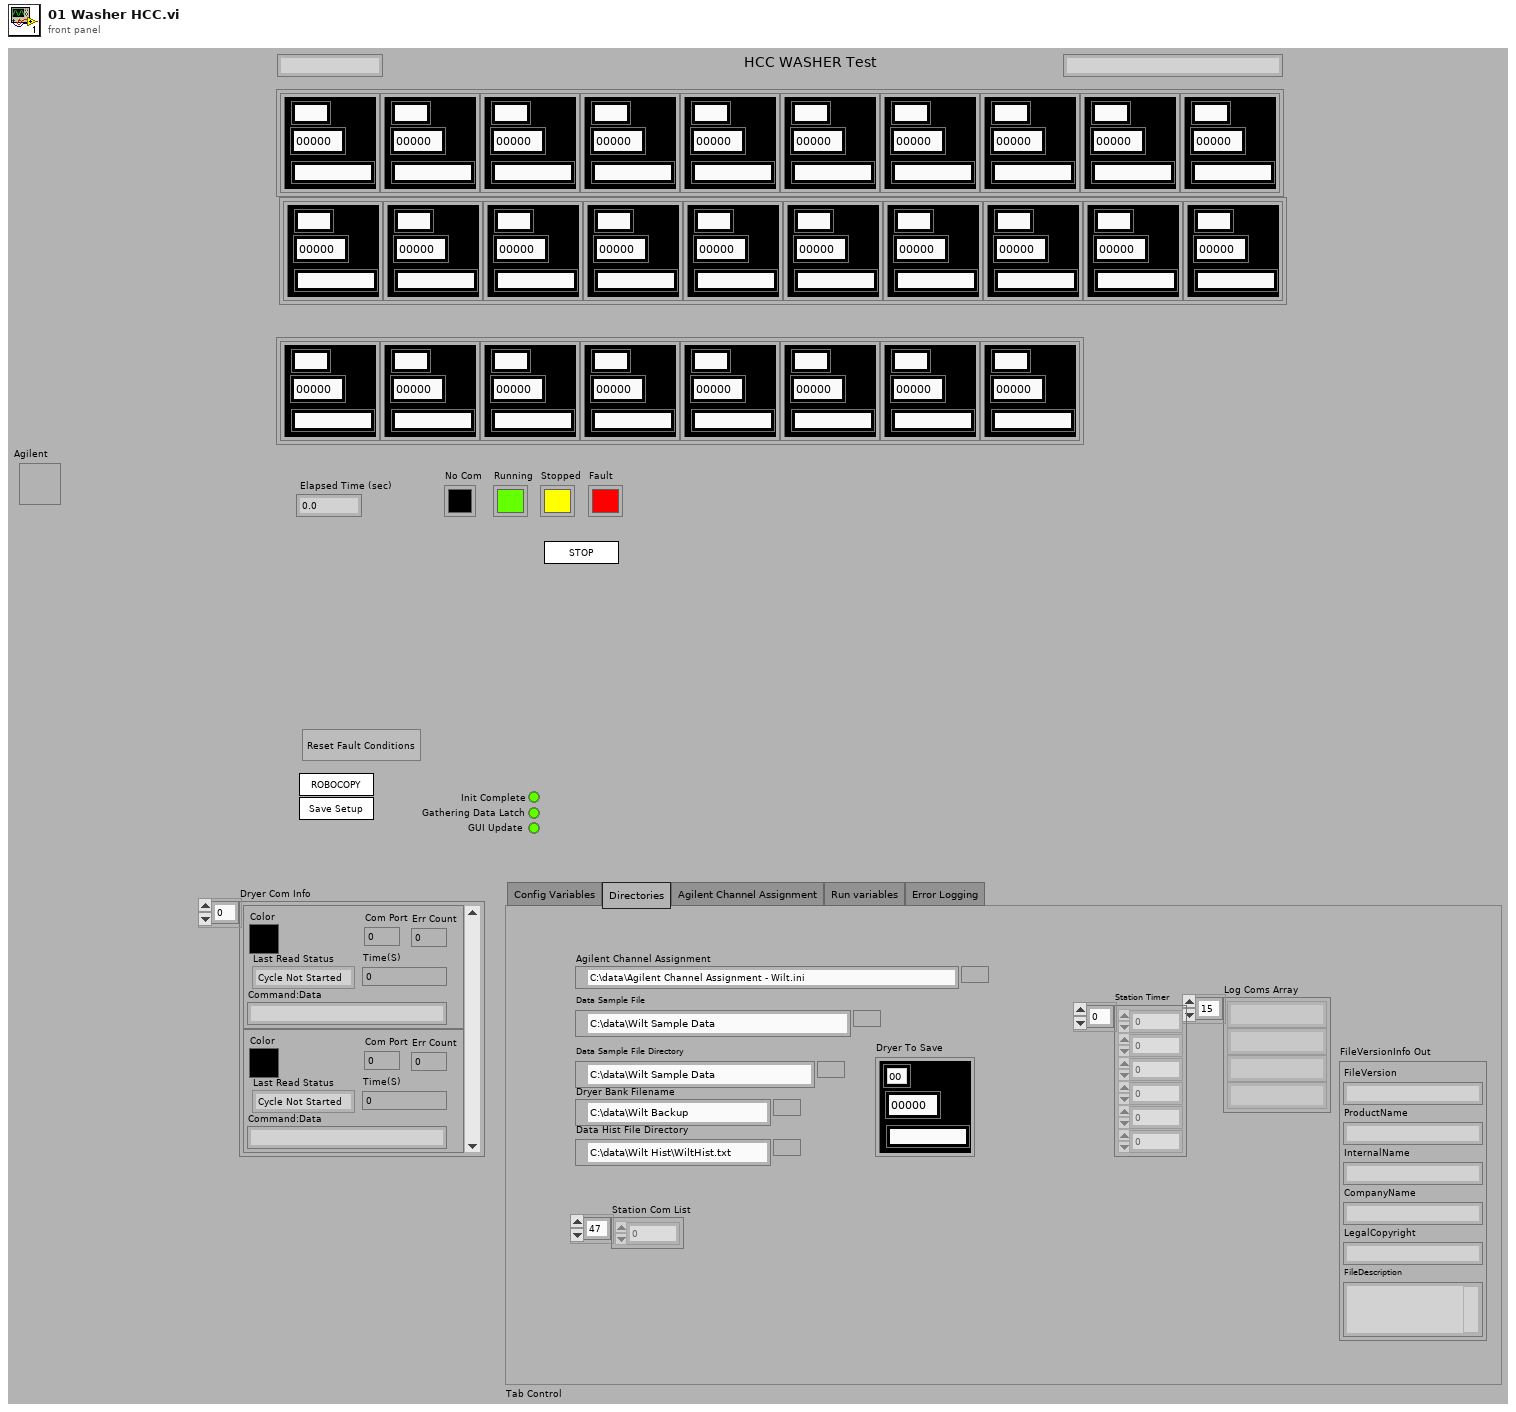
[diagram p1: front panel]
types:
  T1 = typedef "Semaphore RefNum" = refnum<k1>
  T2 = typedef "Dryer Com Port Info.ctl" = cluster{"Color":u32, "Last Read Status":T3, "Command:Data":string, "Com Port":u8, "Time(S)":dbl, "Err Count":u8}
  T3 = typedef "Dryer Status Ctrl.ctl" = enum16{"Cycle Not Started", "Cycle Running", "Paused", "Cycle Completed", "Eval Mode Entered", "Err"}
  T4 = typedef "Washer.ctl" = cluster{"Serial Number":string, "Cycle Count":i32, "Station Number":string, "Dryer Details":T5, "Sample Record(t, CC, ASCII, Status ) ":string[], "Hist Record(Cycle Count, t-comp) ":string[][], "Status Color":u32, "Com Port":u8, "Bad Com Count":i32, "Boolean":bool}
  T5 = typedef "Dryer Details.ctl" = cluster{"Station":string, "Cycle Count":string, "Status":string, "Debug ASCII":string, "Notes":string, "File: Current Cycle":string, "Serial Number":string, "Total Time On":string, "TR Number":string, "File: Historic Data":string}
  T6 = enum32{"Config Variables", "Directories", "Agilent Channel Assignment", "Run variables", "Error Logging"}
  T7 = typedef "Dryer.ctl" = cluster{"Serial Number":string, "Cycle Count":i32, "Station Number":u8, "Dryer Details":T5, "Sample Record(t, CC, Tc, ASCII, Status, L1,L2,Trmb,V{,V2,SW} ) ":string[], "Hist Record(Cycle Count, t-comp,L1max, L2max, Tmax) ":string[][], "Status Color":u32, "Boolean":bool, "Com Port":u8, "Bad Com Count":i32}
  T8 = typedef "FileVersionInformation.ctl" = cluster{"FileVersion":string, "ProductName":string, "InternalName":string, "CompanyName":string, "LegalCopyright":string, "FileDescription":string}
  T9 = typedef "Agilent Channel Definition.ctl" = cluster{"Channel":string, "Station":string, "Label":string, "Agilent Station":string}
  T10 = typedef "Dryer Test State.ctl" = enum16{"No SN", "Wait Com", "Wait to Start", "Watering", "Drying", "Cooldown", "Paused", "Temp Fault"}
  T11 = enum16{"Write History", "Write Sample Data", "Write Dryer Bank", "Read Dryer Bank", "Read Sample History"}
  T12 = cluster{"Data Sample File":path, "Data Hist File Directory":path, "Data Sample File Directory":path, "Agilent Read Refs":refnum<visa-resource-name>[], "All Confgured Com Array":u8[], "Elapsed Time (sec)":dbl, "GUI Aisle Bot":T4[], "GUI Aisle Mid":T4[], "GUI Aisle Top":T4[], "Last Save Hour":string, "Save Bool":bool}
  T13 = enum32{"invalid app kind", "Development System", "Run Time System", "Student Edition", "Embedded LabVIEW", "Evaluation", "Custom"}
  T14 = typedef "GEA2 Dryer Interface Ctrl.ctl" = enum16{"Init Com Port", "SendCMD", "ReadPort", "Close Port", "Simulate Diag Data", "Simulate Dryer", "Send WILT Startup CMDs", "Send Continue CMD", "Read Continuous"}
  T15 = enum32{"Invalid", "Standard", "Closed", "Hidden", "Minimized", "Maximized"}
  T16 = cluster{"Core":cluster{"Current VI Reference":refnum<vi>, "Close Panel on Exit?":bool}, "Agilent Refs":refnum<visa-resource-name>[], "GUI Aisle Top":T4[], "GUI Aisle Mid":T4[], "GUI Aisle Bot":T4[], "Station Timer":dbl[], "Station Test State":T10[], "Saved Test State":T10[], "Dryer Bank Filename":path, "Station Com List":u8[]}
  T17 = cluster{"Current VI Reference":refnum<vi>, "Close Panel on Exit?":bool}
  T18 = typedef "Update Wilt GUI Control.ctl" = enum16{"Init Station Number", "Update Detail Data", "Update Status", "Init Com Port Num", "Update Sample Info"}
  T19 = enum16{"Write History", "Write Sample Data", "Write Dryer Bank", "Read Dryer Bank"}
  T20 = cluster{"GUI Aisle Bot":T4[], "GUI Aisle Mid":T4[], "GUI Aisle Top":T4[], "Dryer To Save":T7}
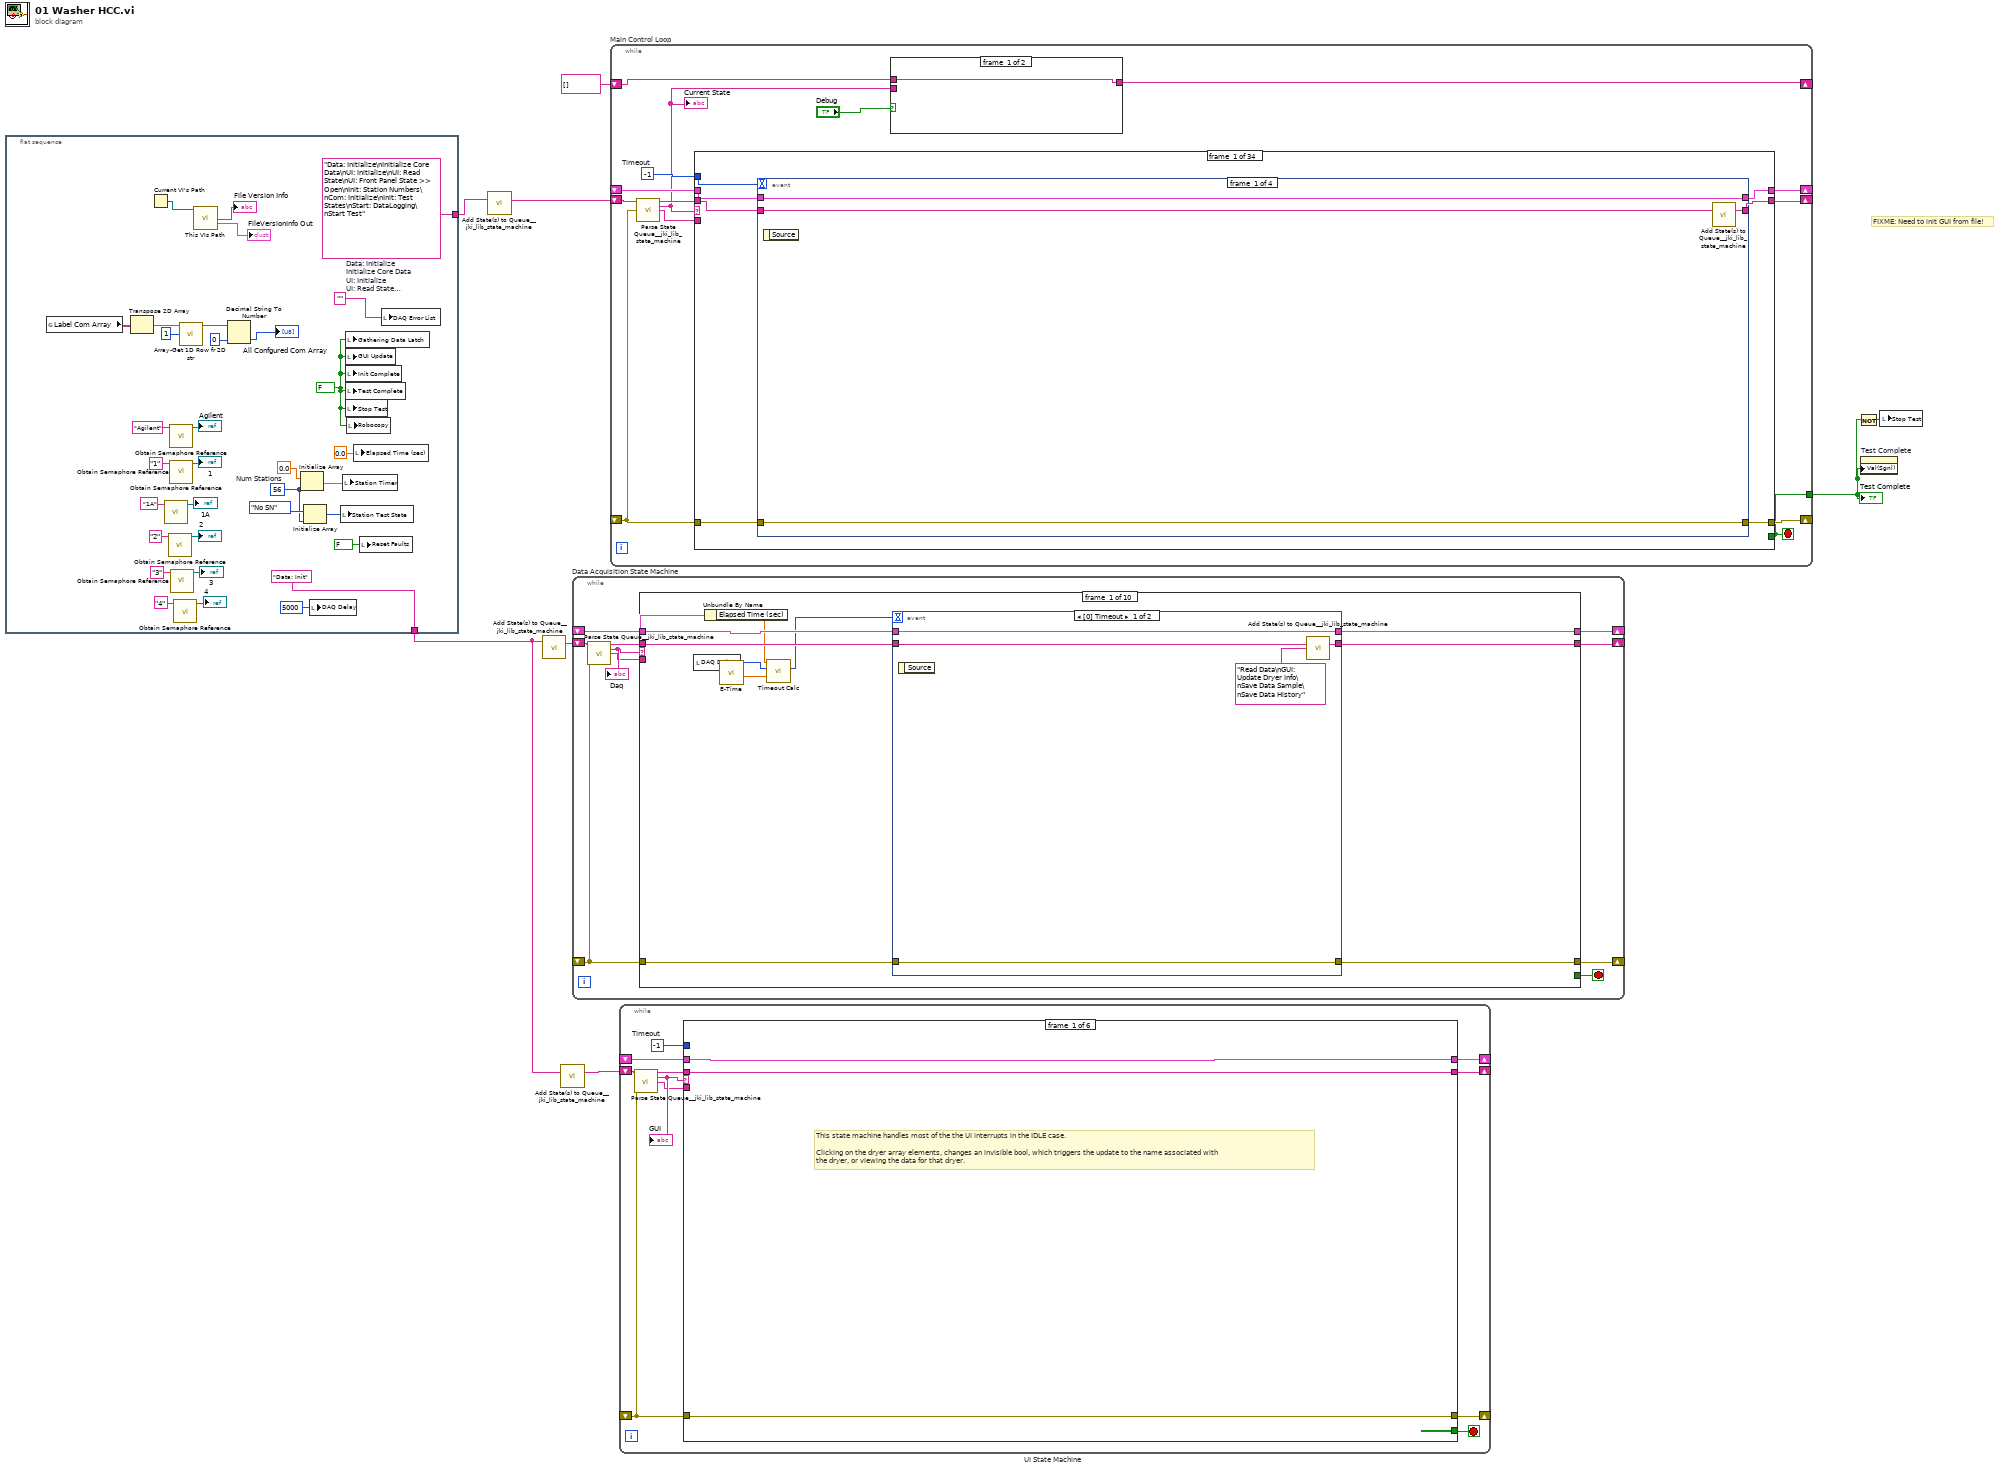
[diagram p0: block diagram]
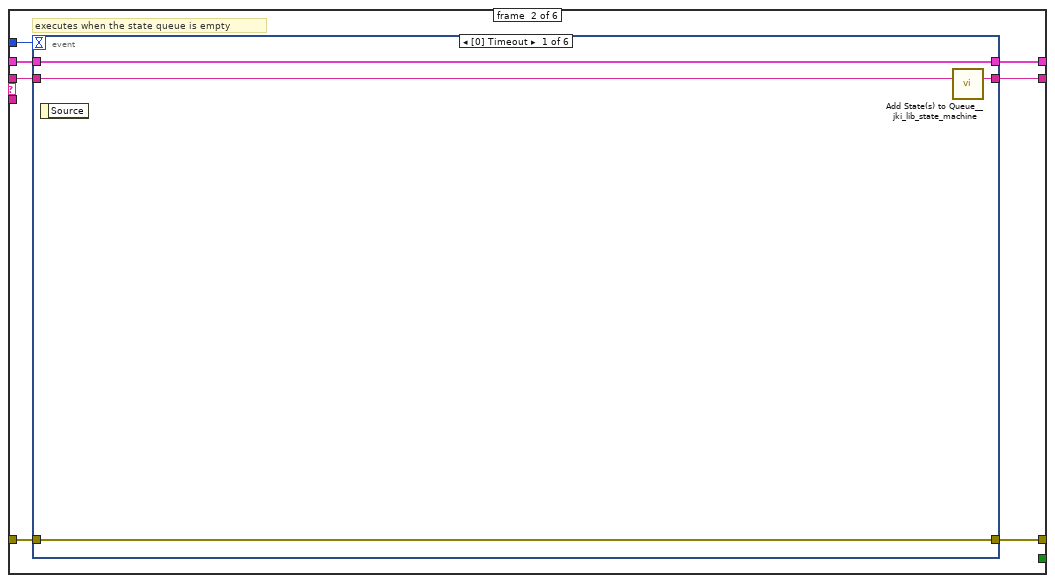
[diagram p2: hidden frame]
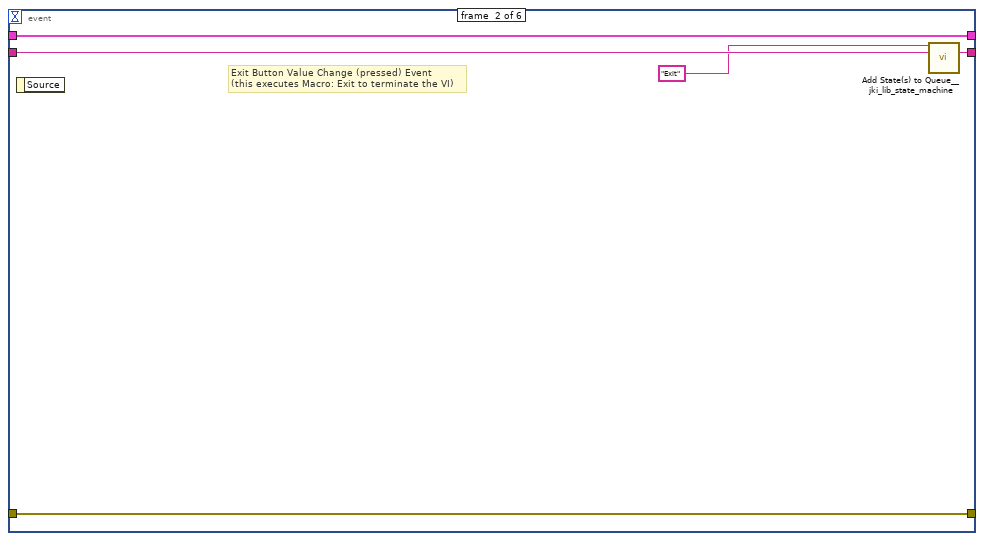
[diagram p3: hidden frame]
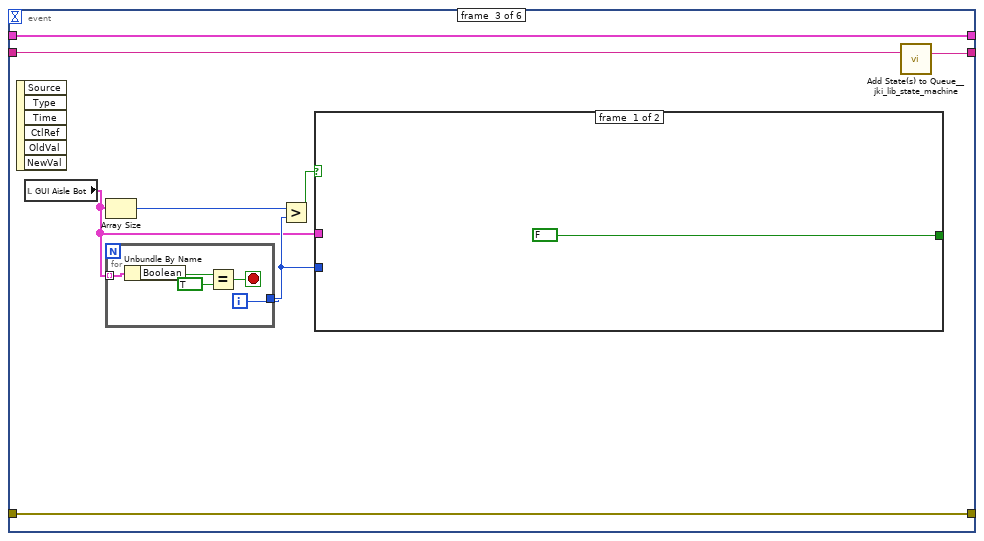
[diagram p4: hidden frame]
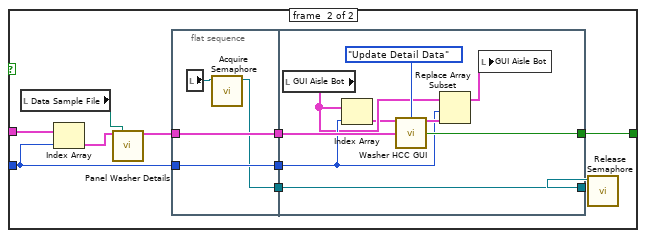
[diagram p5: hidden frame]
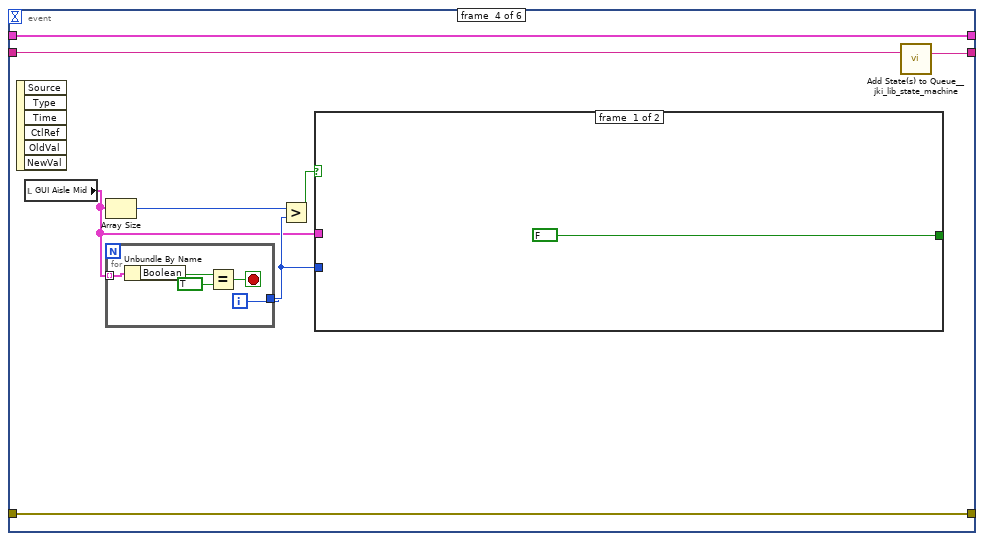
[diagram p6: hidden frame]
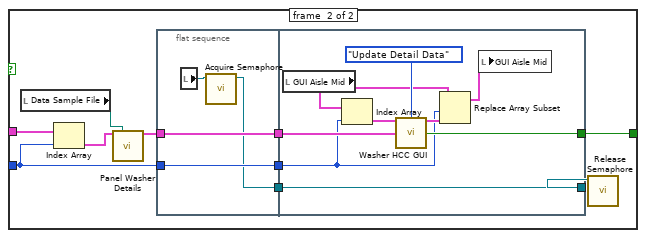
[diagram p7: hidden frame]
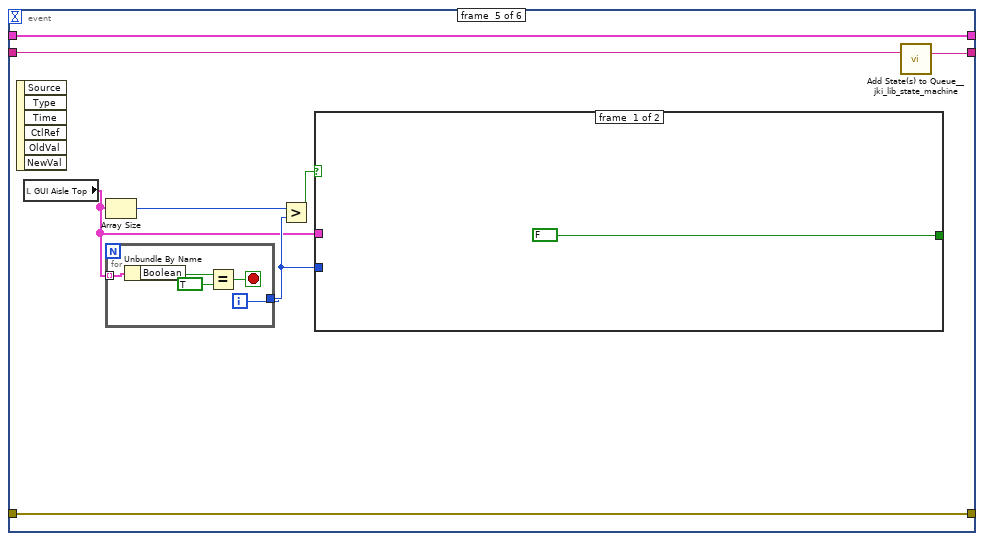
[diagram p8: hidden frame]
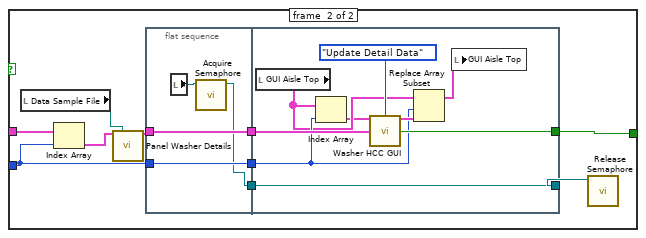
[diagram p9: hidden frame]
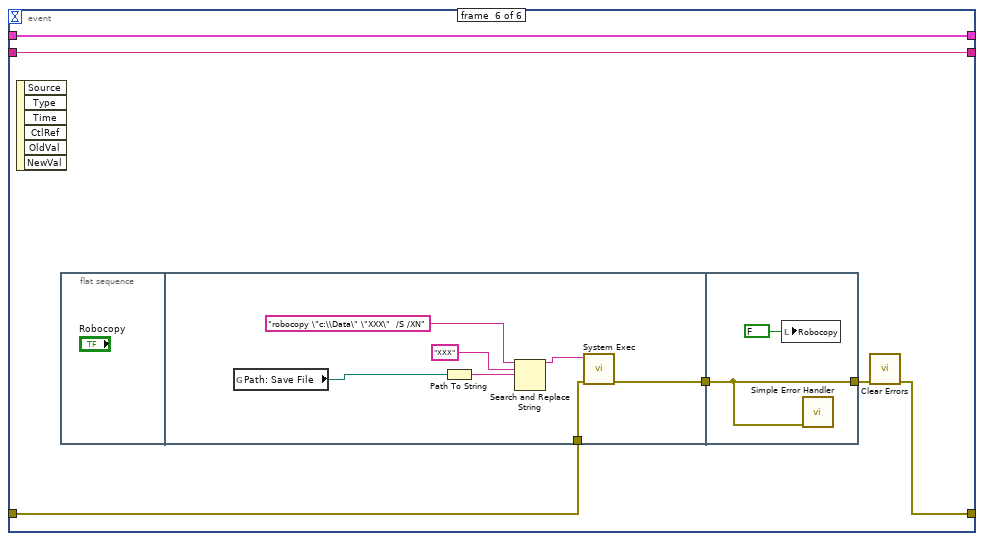
[diagram p10: hidden frame]
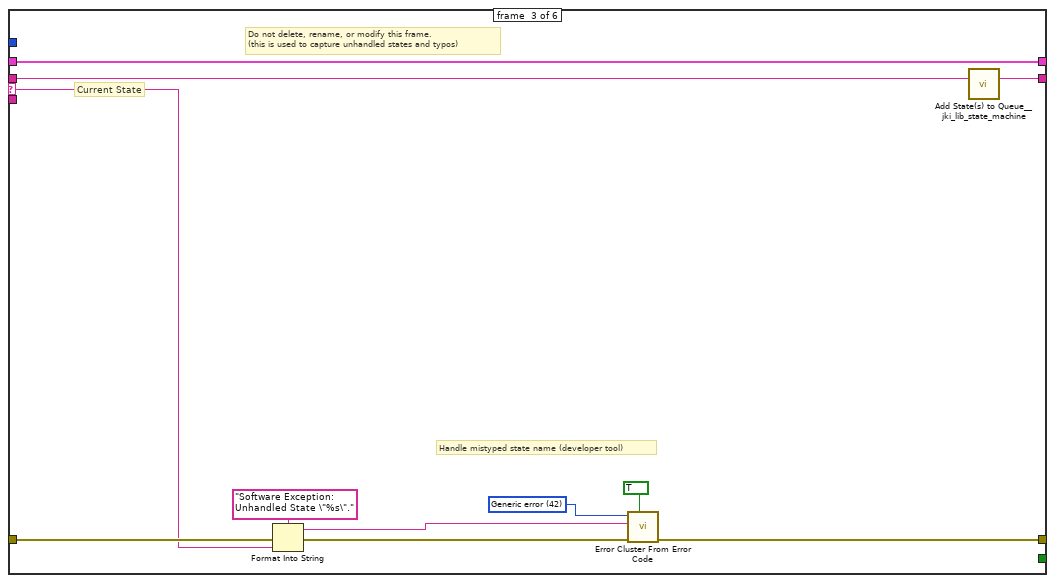
[diagram p11: hidden frame]
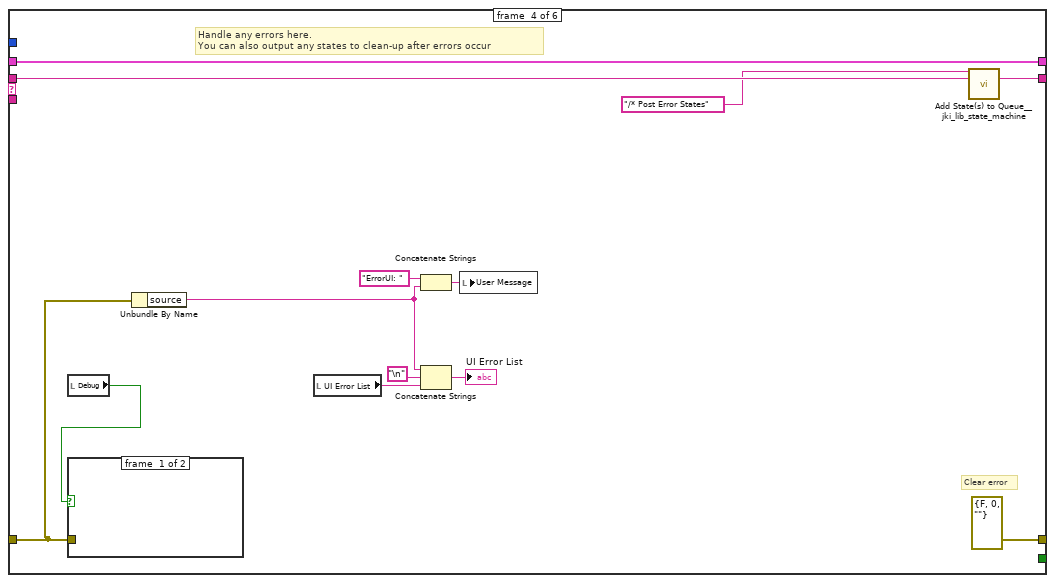
[diagram p12: hidden frame]
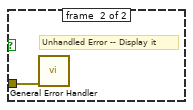
[diagram p13: hidden frame]
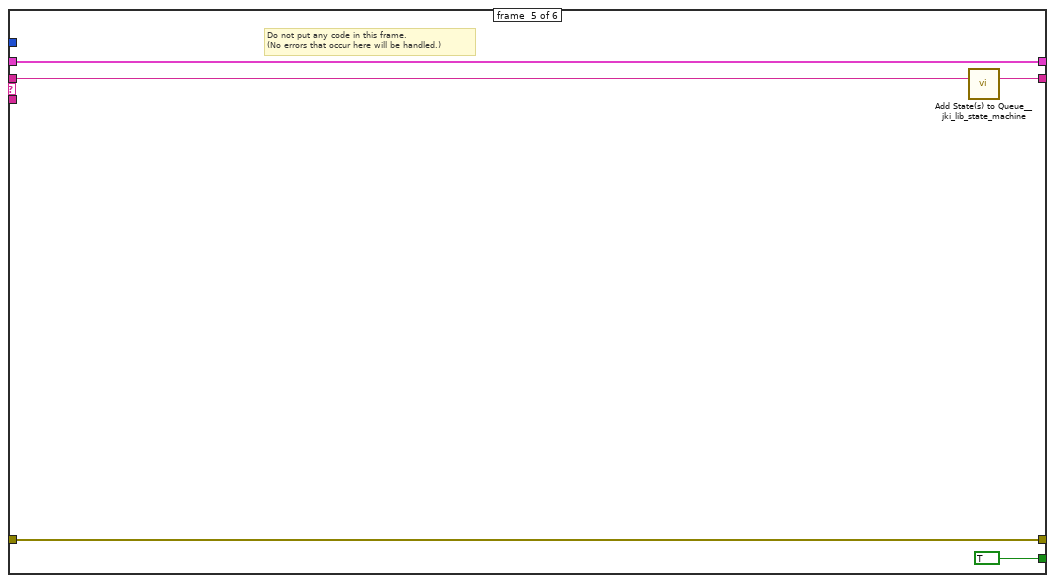
[diagram p14: hidden frame]
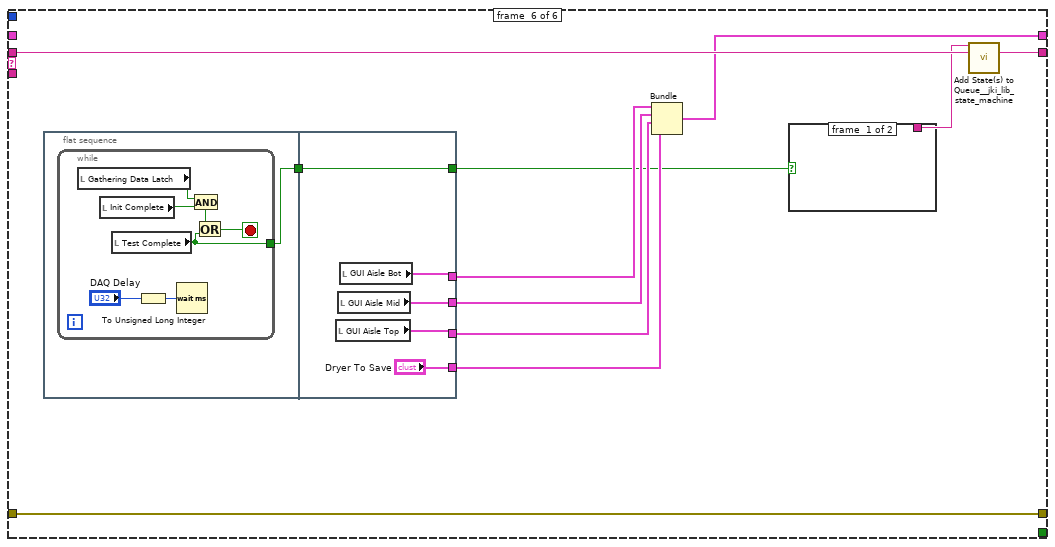
[diagram p15: hidden frame]
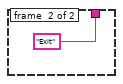
[diagram p16: hidden frame]
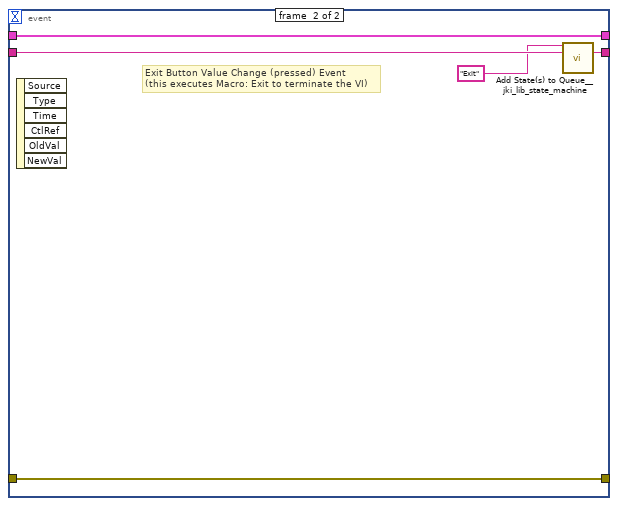
[diagram p17: hidden frame]
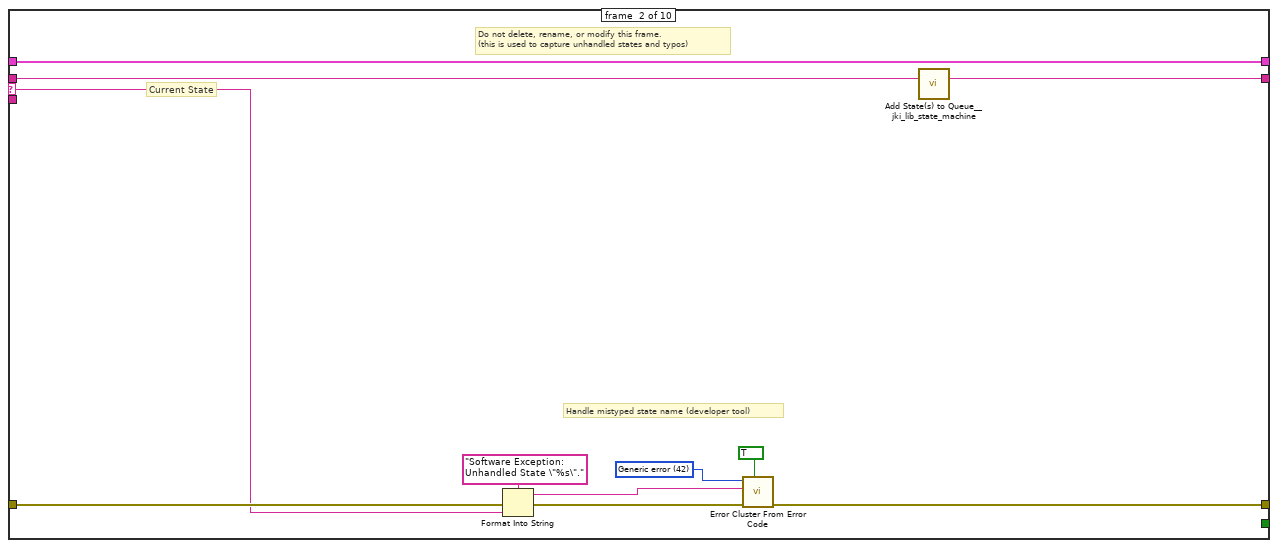
[diagram p18: hidden frame]
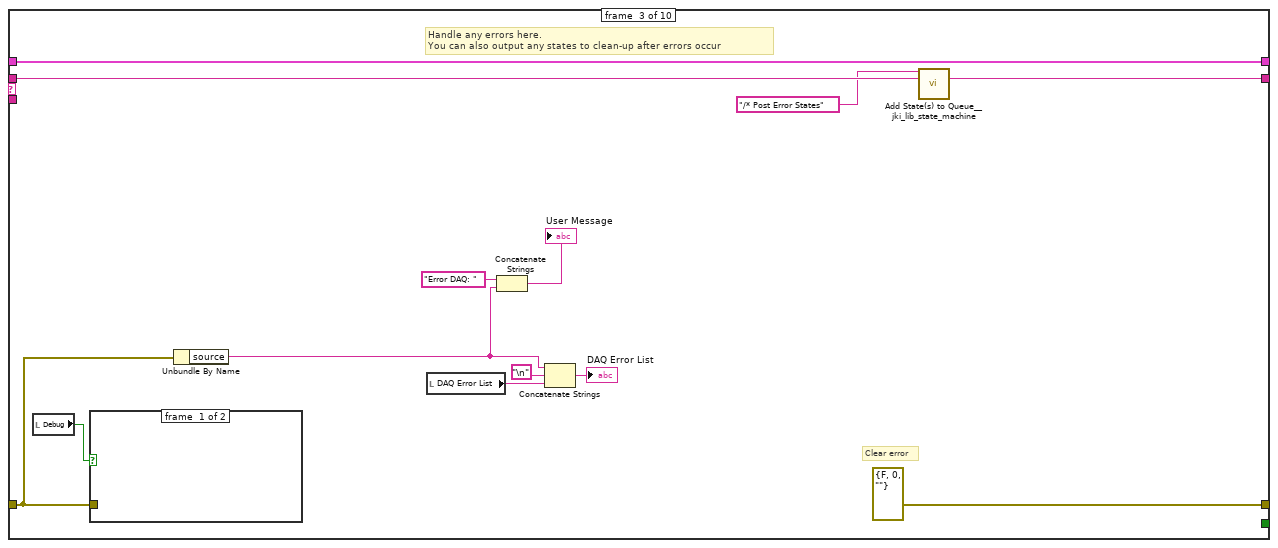
[diagram p19: hidden frame]
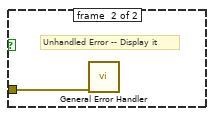
[diagram p20: hidden frame]
diagram:
  # "FIXME: Need to init GUI from file!"
  n1 = flat-sequence {
    tunnel: [w39] -> w7
    tunnel: ["Data: Init"] -> w2
    frame #0 {
      w24 = 56  # Num Stations
      w39 = "Data: Initialize\nInitialize Core Data\nUI: Initialize\nUI: Read State\nUI: Front Panel State >> Open\nInit: Station Numbers\nCom: Initialize\nInit: Test States\nStart: DataLogging\nStart Test"  # Data: Initialize Initialize Core Data UI: Initialize UI: Read State UI: Front Panel State >> Open Init: Station Numbers Com: Initialize Init: Test States Start: DataLogging Start Test
      w22 = FALSE ("Init Complete")
      n2 = global read "Globals HCC.vi" "Label Com Array"() -> (w12:string[][])
      n3 = Transpose 2D Array(2D array=w12) -> (transposed array=w11:string[][])
      n4 = Current VI's Path() -> (path=w19:path)
      n5 = call <vilib>:"Obtain Semaphore Reference.vi"("name (unnamed)"="1A") -> ("semaphore"=→"1A":T1)  [unwired: 4 in, 2 out]
      n6 = call <vilib>:"Obtain Semaphore Reference.vi"("name (unnamed)"="2") -> ("semaphore"=→"2":T1)  [unwired: 4 in, 2 out]
      n7 = call <vilib>:"Obtain Semaphore Reference.vi"("name (unnamed)"="Agilent") -> ("semaphore"=→"Agilent":T1)  [unwired: 4 in, 2 out]
      n8 = call <vilib>:"Obtain Semaphore Reference.vi"("name (unnamed)"="1") -> ("semaphore"=→"1":T1)  [unwired: 4 in, 2 out]
      n9 = call <vilib>:"Obtain Semaphore Reference.vi"("name (unnamed)"="3") -> ("semaphore"=→"3":T1)  [unwired: 4 in, 2 out]
      n10 = call <vilib>:"Obtain Semaphore Reference.vi"("name (unnamed)"="4") -> ("semaphore"=→"4":T1)  [unwired: 4 in, 2 out]
      n11 = call "Array-Get 1D Row fr 2D str.vi"("all rows"=w11, "row index"=1) -> ("row"=w13:string[])  [unwired: 13 in]
      n12 = call "This VIs Path.vi"("path"=w19) -> ("File Version Info"=→"File Version Info":string, "FileVersionInfo Out"=→"FileVersionInfo Out":T8)  [unwired: 10 in, 3 out]
      n13 = Decimal String To Number(string=w13, default (0L)=u8 0 ("default (0 I32)")) -> (number=→"All Confgured Com Array":u8[])  [unwired: 1 in, 1 out]
      n14 = Initialize Array(0.0 ("element"), w24) -> (w26:dbl[])
      n15 = Initialize Array(Dryer_Test_State."No SN" ("Test State"), w24) -> (w23:T10[])
      n16 = local write "DAQ Delay"(u32 5000 ("DAQ Delay")) -> ()
      n17 = local write "Station Test State"(w23) -> ()
      n18 = local write "Station Timer"(w26) -> ()
      n19 = local write "Gathering Data Latch"(w22) -> ()
      n20 = local write "GUI Update"(w22) -> ()
      n21 = local write "Init Complete"(w22) -> ()
      n22 = local write "Test Complete"(w22) -> ()
      n23 = local write "Stop Test"(w22) -> ()
      n24 = local write "Robocopy"(w22) -> ()
      n25 = local write "Elapsed Time (sec)"(0.0 ("Elapsed Time (sec)")) -> ()
      n26 = local write "Reset Faults"(FALSE ("Reset Faults")) -> ()
      n27 = local write "DAQ Error List"("" ("User Notice")) -> ()
    }
  }
  n28 = call <vilib>:"Add State(s) to Queue__jki_lib_state_machine.vi"("State(s) in (\"\")"=w7) -> ("States Out"=w8:string)  [unwired: 14 in]
  n29 = call <vilib>:"Add State(s) to Queue__jki_lib_state_machine.vi"("State(s) in (\"\")"=w2) -> ("States Out"=w6:string)  [unwired: 14 in]
  n30 = call <vilib>:"Add State(s) to Queue__jki_lib_state_machine.vi"("State(s) in (\"\")"=w2) -> ("States Out"=w5:string)  [unwired: 14 in]
  n31 = while "Data Acquisition State Machine" {
    shift-right: [w44] -> _
    shift-left: _ -> [w43]
    shift-right: [w47] -> _
    shift-left: _ -> [w42]
    shift-right: [w46] -> _
    shift-left: w6 -> [w48]
    stop <- w45 stop-if-true
    n32 = call <vilib>:"Parse State Queue__jki_lib_state_machine.vi"("State Queue"=w48, "Error In (no error)"=w42) -> ("Remaining States"=w50:string, "Current State"=w51:string, "Arguments"=w49:string)  [unwired: 11 in]
    "Daq" <- w51
    n33 = case shown="\"Save Data Sample\"" w51 {
      selector: w51 -> [_ w72 _ _ _ _ _ _ _ _]
      tunnel: w50 -> [w61 w76 w95 w101 w105 w123 w161 w169 w239 w244]
      tunnel: w49 -> [_ _ _ _ _ _ _ _ _ _]
      tunnel: w43 -> [w56 w74 w92 w99 w102 _ w157 w168 w230 w242]
      tunnel: [w59 w78 errorcluster {"status"=FALSE, "code"=0, "source"=""} ("error out") w98 w103 w121 w154 w170 w231 w240] -> w47
      tunnel: w42 -> [w58 w77 w89 w98 w103 w121 w158 w170 w232 w240]
      tunnel: [w60 w75 w94 w100 w104 w122 w160 w172 w238 w243] -> w46
      tunnel: [_ _ _ TRUE _ _ _ _ _ _] -> w45
      tunnel: [w57 w74 w92 w99 w102 w120 w156 w171 w229 w242] -> w44
      frame #0 {
        n34 = local read "DAQ Delay"() -> (w53:u32)
        n35 = Unbundle By Name(w56) -> ("Elapsed Time (sec)"=w55:dbl)
        n36 = call "E-Time.vi"() -> ("Elapsed Time (sec)"=w54:dbl)  [unwired: 9 in, 2 out]
        n37 = call "Timeout Calc.vi"("Complete time"=w54, "Gather Data Period"=w53, "Start Time"=w55) -> ("Delay Time"=w52:i32)  [unwired: 8 in]
        n38 = event shown="[0] Timeout" {
          selector: _ -> [_ _]
          dyn-events: _ -> [_ _]
          timeout: w52 -> [_ _]
          tunnel: w61 -> [w66 w71]
          tunnel: [w65 w70] -> w60
          tunnel: w56 -> [w63 w68]
          tunnel: [w64 w69] -> w59
          tunnel: w58 -> [w64 w69]
          tunnel: [w63 w68] -> w57
          event #0 {
            n39 = event-data() -> ()  [unwired: 1 in, 1 out]
            n40 = call <vilib>:"Add State(s) to Queue__jki_lib_state_machine.vi"("State(s) in (\"\")"=w66, "State(s) at Back (\"\")"="Read Data\nGUI: Update Dryer Info\nSave Data Sample\nSave Data History") -> ("States Out"=w65:string)  [unwired: 13 in]
          }
          event #1 {
            # "Exit Button Value Change (pressed) Event\n(this executes Macro: Exit to terminate the VI)"
            n41 = event-data() -> ()  [unwired: 1 in, 6 out]
            n42 = call <vilib>:"Add State(s) to Queue__jki_lib_state_machine.vi"("State(s) in Front (\"\")"="Exit", "State(s) in (\"\")"=w71) -> ("States Out"=w70:string)  [unwired: 13 in]
          }
        }
      }
      frame #1 {
        w81 = 42 items=["No error", "Argument error", "Memory is full", "Out of zone", "End of file", "File already open", "Generic file I/O error", "File not found", "File permission error", "Disk is full", "Duplicate path", "Too many files open", "System feature not enabled", "Resource file not found", "Cannot add resource", "Resource not found", "Image not found", "Image memory error", "Pen does not exist", "Config type invalid", "Config token not found", "Config parse error", "Config memory error", "Bad external code format", "Bad external code offset", "External code not present", "Null window", "Destroy window error", "Null menu", "Print aborted", "Bad print record", "Print driver error", "Windows error during printing", "Memory error during printing", "Print dialog error", "Generic print error", "Invalid device refnum", "Device not found", "Device parameter error", "Device unit error", "Cannot open device", "Device call aborted", "Generic error", "Cancelled by user", "Object ID too low", "Object ID too high", "Object not in heap", "Unknown heap", "Unknown object (invalid DefProc)", "Unknown object (DefProc not in table)", "Message out of range", "Invalid (null) method", "Unknown message", "Manager call not supported", "Bad address", "Network operation in progress", "Network operation timed out", "Connection is busy", "Network attribute not supported", "Network error", "Address in use", "System out of memory", "Connection aborted", "Connection refused", "Not connected", "Already connected", "Connection closed", "Initialization error (interapplication manager)", "Bad occurrence", "Wait on unbound occurrence handler", "Occurrence queue overflow", "Datalog type conflict", "Unused", "Unrecognized type (interapplication manager)", "Memory corrupt", "Failed to make temporary DLL", "Old CIN version", "Drag socket not found", "Failed to load drop-object", "Failed to register OLE object", "Failed to release OLE object", "Format specifier type mismatch", "Unknown format specifier", "Too few format specifiers", "Too many format specifiers", "Scan failed", "Newer CIN version", "Error converting to variant", "Runtime menu error", "Password tampered", "Variant attribute not found", "Incompatible variant data type", "Event data is not available", "Event Store is not present", "Occurrence is not found", "Event Queue is not created", "Event info is not available", "Refnum passed is NULL", "Error retrieving Class GUID", "Error retrieving CoClass GUID", "Error retrieving TypeLib GUID.", "Bad built application magic bytes.", "Specific driver is different from the specific driver associated with the Logical Name.", "There is no session opened to the class driver.", "Max Error", "MAX - Error with config objects", "MAX - Error loading configuration", "MAX - Group not supported"]
        # "Current State"
        # "Do not delete, rename, or modify this frame.\n(this is used to capture unhandled states and typos)"
        # "Handle mistyped state name (developer tool)"
        n43 = Format Into String(format string="Software Exception: Unhandled State \"%s\"." ("message"), error in=w77, w72) -> (resulting string=w80:string, error out=w79:errorcluster)  [unwired: 1 in]
        n44 = call <vilib>:"Error Cluster From Error Code.vi"("show call chain? (False)"=TRUE, "error in (no error)"=w79, "error message (\"\")"=w80, "error code (0)"=w81) -> ("error out"=w78:errorcluster)  [unwired: 5 in]
        n45 = call <vilib>:"Add State(s) to Queue__jki_lib_state_machine.vi"("State(s) in (\"\")"=w76) -> ("States Out"=w75:string)  [unwired: 14 in]
      }
      frame #2 {
        # "Handle any errors here.\nYou can also output any states to clean-up after errors occur"
        # "Clear error"
        n46 = local read "Debug"() -> (w83:bool)
        n47 = case shown="True" w83 {
          tunnel: w89 -> [_ w96]
          frame #0 {
          }
          frame #1 {
            # "Unhandled Error -- Display it"
            n48 = call <vilib>:"General Error Handler.vi"("error in (no error)"=w96) -> ()  [unwired: 10 in, 5 out]
          }
        }
        n49 = Unbundle By Name(w89) -> ("source"=w86:string)
        n50 = local read "DAQ Error List"() -> (w84:string)
        n51 = Concatenate Strings("Error DAQ: " ("string"), w86) -> (→"User Message":string)
        n52 = Concatenate Strings(w86, "\n", w84) -> (→"DAQ Error List":string)
        n53 = call <vilib>:"Add State(s) to Queue__jki_lib_state_machine.vi"("State(s) in Front (\"\")"="/* Post Error States", "State(s) in (\"\")"=w95) -> ("States Out"=w94:string)  [unwired: 13 in]
      }
      frame #3 {
        # "Do not put any code in this frame.\n(No errors that occur here will be handled.)"
        n54 = call <vilib>:"Add State(s) to Queue__jki_lib_state_machine.vi"("State(s) in (\"\")"=w101) -> ("States Out"=w100:string)  [unwired: 14 in]
      }
      frame #4 {
        # "Template Separator\n(You can make a copy of, or modify, this frame)"
        n55 = call <vilib>:"Add State(s) to Queue__jki_lib_state_machine.vi"("State(s) in (\"\")"=w105) -> ("States Out"=w104:string)  [unwired: 14 in]
      }
      frame #5 {
        # "Data Log Time"
        # "Template Separator\n(You can make a copy of, or modify, this frame)"
        n56 = flat-sequence {
          tunnel: [w125] -> w115
          tunnel: [w138] -> w119
          tunnel: [w141] -> w118
          tunnel: [w140] -> w117
          tunnel: [w139] -> w116
          tunnel: w115 -> [w139]
          tunnel: [w133] -> w113
          tunnel: [w132] -> w112
          tunnel: [w131] -> w111
          tunnel: ["Data Hist File Directory"] -> w110
          tunnel: ["Data Sample File Directory"] -> w109
          tunnel: [w135] -> w108
          tunnel: ["Data Sample File"] -> w107
          tunnel: [w130] -> w106
          frame #0 {
            n57 = while {
              tunnel: [w126] -> w125
              stop <- w128 stop-if-true
              n58 = local read "DAQ Delay"() -> (w127:u32)
              n59 = local read "Test Complete"() -> (w126:bool)
              n60 = local read "Init Complete"() -> (w129:bool)
              n61 = Wait (ms)(milliseconds to wait=w127) -> ()  [unwired: 1 out]
              n62 = Or(x=w129, y=w126) -> (x .or. y?=w128:bool)
            }
          }
          frame #1 {
            w130 = FALSE  # Save Bool
            w135 = "%H"  # Last Save Hour
            n63 = local read "GUI Aisle Top"() -> (w131:T4[])
            n64 = local read "GUI Aisle Mid"() -> (w132:T4[])
            n65 = local read "GUI Aisle Bot"() -> (w133:T4[])
            n66 = local read "All Confgured Com Array"() -> (w141:u8[])
            n67 = local read "Agilent Read Refs"() -> (w138:refnum<visa-resource-name>[])
            n68 = call "E-Time.vi"() -> ("Elapsed Time (sec)"=w140:dbl)  [unwired: 9 in, 2 out]
          }
        }
        n69 = case shown="False" w116 {
          tunnel: [_ "Exit" ("State(s) in Front (\"\")")] -> w114
          frame #0 {
          }
          frame #1 {
          }
        }
        n70 = Bundle("Data Sample File"=w107, "Data Hist File Directory"=w110, "Data Sample File Directory"=w109, "Agilent Read Refs"=w119, "All Confgured Com Array"=w118, "Elapsed Time (sec)"=w117, "GUI Aisle Bot"=w113, "GUI Aisle Mid"=w112, "GUI Aisle Top"=w111, "Last Save Hour"=w108, "Save Bool"=w106) -> (w120:T12)  [unwired: 1 in]
        n71 = call <vilib>:"Add State(s) to Queue__jki_lib_state_machine.vi"("State(s) in Front (\"\")"=w114, "State(s) in (\"\")"=w123) -> ("States Out"=w122:string)  [unwired: 13 in]
      }
      frame #6 {
        # "SW set >1e6 values to 1000."
        # "Gathers all data:"
        n72 = Unbundle By Name(w157) -> ("Agilent Read Refs"=w159:refnum<visa-resource-name>[], "All Confgured Com Array"=w152:u8[])
        n73 = local read "Dryer Com Info"() -> (w149:T2[])
        n74 = call "E-Time.vi"("error in (no error)"=w158) -> ("error out"=w153:errorcluster, "Elapsed Time (sec)"=w155:dbl)  [unwired: 8 in, 1 out]
        "Elapsed Time (sec)" <- w155
        n75 = local read "Agilent"() -> (w144:T1)
        n76 = To Unsigned Byte Integer(number=w152) -> (unsigned 8bit integer=w145:u8[])
        n77 = call "Agilent Read 5 Units.vi"("Agilent Refs"=w159, "error in (no error)"=w153, "Agilent"=w144) -> ("All Agilent Data"=w147:dbl[], "error out"=→"Agilent Read Errors":errorcluster)  [unwired: 15 in]
        n78 = call "Read All Washers.vi"("Com Array"=w145, "Status Array In"=w149, "error in (no error)"=w153) -> ("Log Coms Array"=→"Log Coms Array":string[], "Status Array Out"=→"Dryer Com Info":T2[], "error out"=w154:errorcluster)  [unwired: 9 in, 1 out]
        n79 = for {
          tunnel: w147 -> [w165] mode=indexing
          tunnel: [w164] -> w146 mode=indexing
          tunnel: 1000.0 ("t") -> [w163]
          tunnel: 1000000.0 ("y") -> [w162]
          n80 = Greater?(x=w165, y=w162) -> (0:w166:bool)
          n81 = Select(t=w163, s=w166, f=w165) -> (s? t:f=w164:dbl)
        }
        "Current Agilent Data" <- w146
        n82 = Bundle By Name(cluster=w157, "Elapsed Time (sec)"=w155) -> (w156:T12)
        n83 = case shown="No Error" w154 {
          frame #0 {
            w167 = TRUE
            n84 = property on="Gathering Data Latch" class="Bool (strict)"("Val(Sgnl)"=w167) -> ()  [unwired: 2 in, 2 out]
            "Gathering Data Latch" <- w167
          }
          frame #1 {
          }
        }
        n85 = call <vilib>:"Add State(s) to Queue__jki_lib_state_machine.vi"("State(s) in (\"\")"=w161) -> ("States Out"=w160:string)  [unwired: 14 in]
      }
      frame #7 {
        # "Upadate Aisle Info with Agilent Data."
        n86 = local read "Current Agilent Data"() -> (w174:dbl[])
        n87 = flat-sequence {
          tunnel: [w221] -> w175
          frame #0 {
            n88 = local read "Agilent Station Data Index Array"() -> (w221:i32[][])
            n89 = local write "GUI Update"(FALSE ("GUI Updatge")) -> ()
          }
        }
        n90 = local read "Dryer Com Info"() -> (w173:T2[])
        n91 = flat-sequence {
          tunnel: w173 -> [w214]
          tunnel: [w214] -> w190
          tunnel: [w212] -> w189
          tunnel: w174 -> [_]
          tunnel: w175 -> [_]
          tunnel: w190 -> [w217]
          tunnel: [w216] -> w188
          tunnel: w189 -> [w216]
          tunnel: [w215] -> w181
          tunnel: w188 -> [w220]
          tunnel: [w219] -> w176
          frame #0 {
            n92 = local read "4"() -> (w213:T1)
            n93 = call <vilib>:"Acquire Semaphore.vi"("semaphore"=w213) -> ("semaphore out"=w212:T1)  [unwired: 4 in, 2 out]
          }
          frame #1 {
            n94 = local read "GUI Aisle Top"() -> (w218:T4[])
            n95 = call "Update Washer Records.vi"("GUI Aisle In"=w218, "Dryer Com Info"=w217) -> ("Aisle Array Out"=w215:T4[])  [unwired: 13 in]
            n96 = local write "GUI Aisle Top"(w215) -> ()
          }
          frame #2 {
            n97 = call <vilib>:"Release Semaphore.vi"("semaphore"=w220) -> ("error out"=w219:errorcluster)  [unwired: 5 in, 1 out]
          }
        }
        n98 = flat-sequence {
          tunnel: w173 -> [w205]
          tunnel: [w205] -> w187
          tunnel: [w203] -> w186
          tunnel: w174 -> [_]
          tunnel: w175 -> [_]
          tunnel: w187 -> [w208]
          tunnel: [w207] -> w185
          tunnel: w186 -> [w207]
          tunnel: [w206] -> w180
          tunnel: w185 -> [w211]
          tunnel: [w210] -> w177
          frame #0 {
            n99 = local read "3"() -> (w204:T1)
            n100 = call <vilib>:"Acquire Semaphore.vi"("semaphore"=w204) -> ("semaphore out"=w203:T1)  [unwired: 4 in, 2 out]
          }
          frame #1 {
            n101 = local read "GUI Aisle Mid"() -> (w209:T4[])
            n102 = call "Update Washer Records.vi"("GUI Aisle In"=w209, "Dryer Com Info"=w208) -> ("Aisle Array Out"=w206:T4[])  [unwired: 13 in]
            n103 = local write "GUI Aisle Mid"(w206) -> ()
          }
          frame #2 {
            n104 = call <vilib>:"Release Semaphore.vi"("semaphore"=w211) -> ("error out"=w210:errorcluster)  [unwired: 5 in, 1 out]
          }
        }
        n105 = flat-sequence {
          tunnel: w173 -> [w195]
          tunnel: [w195] -> w184
          tunnel: [w193] -> w183
          tunnel: [w197] -> _
          tunnel: w175 -> [_]
          tunnel: w184 -> [w199]
          tunnel: [w198] -> w182
          tunnel: w183 -> [w198]
          tunnel: w174 -> [w197]
          tunnel: [w196] -> w179
          tunnel: w182 -> [w202]
          tunnel: [w201] -> w178
          frame #0 {
            n106 = local read "2"() -> (w194:T1)
            n107 = call <vilib>:"Acquire Semaphore.vi"("semaphore"=w194) -> ("semaphore out"=w193:T1)  [unwired: 4 in, 2 out]
          }
          frame #1 {
            n108 = local read "GUI Aisle Bot"() -> (w200:T4[])
            n109 = call "Update Washer Records.vi"("GUI Aisle In"=w200, "Dryer Com Info"=w199) -> ("Aisle Array Out"=w196:T4[])  [unwired: 13 in]
            n110 = local write "GUI Aisle Bot"(w196) -> ()
          }
          frame #2 {
            n111 = call <vilib>:"Release Semaphore.vi"("semaphore"=w202) -> ("error out"=w201:errorcluster)  [unwired: 5 in, 1 out]
          }
        }
        n112 = flat-sequence {
          tunnel: w176 -> [_]
          tunnel: [w191] -> _
          tunnel: w177 -> [w191]
          tunnel: w178 -> [_]
          frame #0 {
            "GUI Update" <- TRUE ("GUI Updatge")
          }
        }
        n113 = call <vilib>:"Add State(s) to Queue__jki_lib_state_machine.vi"("State(s) in (\"\")"=w169) -> ("States Out"=w172:string)  [unwired: 14 in]
        n114 = Bundle By Name(cluster=w168, "GUI Aisle Top"=w181, "GUI Aisle Mid"=w180, "GUI Aisle Bot"=w179) -> (w171:T12)
      }
      frame #8 {
        # "Template Separator\n(You can make a copy of, or modify, this frame)"
        n115 = Unbundle By Name(w230) -> ("Data Sample File Directory"=w233:path, "GUI Aisle Bot"=w234:T4[], "GUI Aisle Mid"=w235:T4[], "GUI Aisle Top"=w236:T4[], "Last Save Hour"=w225:string, "Data Sample File"=w228:path)
        n116 = Build Array (concatenate)(w234, w235, w236) -> (w237:T4[])
        n117 = call "File Washer HCC.vi"("Dryer Aisle In"=w237, "Dryer s,h Data Dir"=w233, "RW  Mode"=T11."Write Sample Data", "Last Save Hour"=w225, "error in (no error)"=w232, "Sample Data Current Filename"=w228) -> ("Last Save Hour Out"=w224:string, "Sample Data Current Filename Out"=w227:path, "error out"=w231:errorcluster)  [unwired: 6 in, 1 out]
        n118 = call <vilib>:"Add State(s) to Queue__jki_lib_state_machine.vi"("State(s) in (\"\")"=w239) -> ("States Out"=w238:string)  [unwired: 14 in]
        n119 = Not Equal?(x=w225, y=w224) -> (x != y?=w223:bool)
        n120 = local write "Data Sample File"(w227) -> ()
        n121 = Bundle By Name(cluster=w230, "Last Save Hour"=w224, "Data Sample File"=w227, "Save Bool"=w223) -> (w229:T12)
      }
      frame #9 {
        # "Template Separator\n(You can make a copy of, or modify, this frame)"
        n122 = Unbundle By Name(w242) -> ("Save Bool"=w241:bool)
        n123 = case shown="True" w241 {
          frame #0 {
          }
          frame #1 {
            # "In 3rd state machine."
            # "In first state machine"
            n124 = local write "Save Setup"(TRUE ("Save Setup")) -> ()
            n125 = property on="Robocopy" class="Bool (strict)"("Val(Sgnl)"=TRUE ("Value (Signaling)")) -> ()  [unwired: 2 in, 2 out]
          }
        }
        n126 = call <vilib>:"Add State(s) to Queue__jki_lib_state_machine.vi"("State(s) in (\"\")"=w244) -> ("States Out"=w243:string)  [unwired: 14 in]
      }
    }
  }
  n127 = while "Main Control Loop" {
    shift-right: [w255] -> _
    shift-left: _ -> [w254]
    shift-right: [w257] -> _
    shift-left: _ -> [w252]
    shift-right: [w256] -> _
    shift-left: w8 -> [w258]
    tunnel: [w251] -> w3
    shift-right: [w249] -> _
    shift-left: string[] [] -> [w248]
    stop <- w251 stop-if-true
    w253 = -1  # Timeout
    n128 = call <vilib>:"Parse State Queue__jki_lib_state_machine.vi"("State Queue"=w258, "Error In (no error)"=w252) -> ("Remaining States"=w260:string, "Current State"=w250:string, "Arguments"=w259:string)  [unwired: 11 in]
    "Current State" <- w250
    n129 = case shown="\"Data: Initialize\"" w250 {
      selector: w250 -> [_ _ w297 _ _ _ _ _ _ _ _ w451 _ _ _ _ _ _ _ _ _ _ _ _ _ _ _ _ _ _ _ _ _ _]
      tunnel: w260 -> [w271 w296 w301 w319 w335 w348 w355 w360 w374 w410 w434 w459 w490 w511 w519 w526 w547 w567 w578 w604 w608 w618 w622 w626 w631 w639 w647 w678 w739 w786 w824 w867 w911 w953]
      tunnel: w259 -> [_ _ _ _ _ _ _ _ _ _ _ _ _ _ _ _ _ w562 w572 _ _ _ _ _ _ _ _ _ _ _ _ _ _ _]
      tunnel: w254 -> [w269 w293 w299 w310 w330 w345 w353 w357 _ w407 w428 w456 w488 w508 w517 w524 w545 w565 w574 w601 w605 w615 w619 w623 w628 w636 w644 w665 w736 w778 w819 w863 w908 w950]
      tunnel: [w268 w294 w303 w316 w331 errorcluster {"status"=FALSE, "code"=0, "source"=""} ("error out") w352 w358 w371 w408 w432 w457 w481 w509 w516 w520 w542 w563 w575 w602 w606 w616 w620 w624 w629 w637 w640 w660 w737 w784 w820 w859 w900 w947] -> w257
      tunnel: w252 -> [w267 w294 w302 w316 w332 w337 w352 w358 w371 w408 w432 w455 w485 w509 w516 w521 w543 w564 w576 w602 w606 w616 w620 w624 w629 w637 w640 w676 w737 w784 w820 w859 w903 w947]
      tunnel: [w270 w295 w300 w318 w334 w347 w354 w359 w373 w409 w433 w458 w489 w510 w518 w525 w546 w566 w577 w603 w607 w617 w621 w625 w630 w638 w646 w677 w738 w785 w823 w866 w910 w952] -> w256
      tunnel: [_ _ _ _ _ _ TRUE _ _ _ _ _ _ _ _ _ _ _ _ _ _ _ _ _ _ _ _ _ _ _ _ _ _ _] -> w251
      tunnel: [w266 w293 w299 w317 w330 w345 w353 w357 w372 w407 w427 w456 w488 w508 w517 w524 w545 w565 w574 w601 w605 w615 w619 w623 w628 w636 w643 w664 w735 w783 w818 w862 w907 w949] -> w255
      tunnel: w253 -> [w265 _ _ _ _ _ _ _ _ _ _ _ _ _ _ _ _ _ _ _ _ _ _ _ _ _ _ _ _ _ _ _ _ _]
      frame #0 {
        n130 = event shown="[2] \"Save Setup\": Value Change" {
          selector: _ -> [_ _ _ _]
          dyn-events: _ -> [_ _ _ _]
          timeout: w265 -> [_ _ _ _]
          tunnel: w271 -> [w275 w281 w286 w292]
          tunnel: [w274 w280 w285 w291] -> w270
          tunnel: w269 -> [w272 w278 w283 w289]
          tunnel: [w273 w279 w284 w290] -> w268
          tunnel: w267 -> [w273 w279 w284 w290]
          tunnel: [w272 w278 w283 w289] -> w266
          event #0 {
            n131 = event-data() -> ()  [unwired: 1 in, 1 out]
            n132 = call <vilib>:"Add State(s) to Queue__jki_lib_state_machine.vi"("State(s) in (\"\")"=w275) -> ("States Out"=w274:string)  [unwired: 14 in]
          }
          event #1 {
            # "Exit Button Value Change (pressed) Event\n(this executes Macro: Exit to terminate the VI)"
            n133 = event-data() -> ()  [unwired: 1 in, 1 out]
            n134 = property on="Stop Test" class="Bool (strict)"("Val(Sgnl)"="Stop Test") -> ()  [unwired: 2 in, 2 out]
            n135 = call <vilib>:"Add State(s) to Queue__jki_lib_state_machine.vi"("State(s) in Front (\"\")"="UI: Save Current State\nExit", "State(s) in (\"\")"=w281) -> ("States Out"=w280:string)  [unwired: 13 in]
          }
          event #2 {
            # "Exit Button Value Change (pressed) Event\n(this executes Macro: Exit to terminate the VI)"
            n136 = event-data() -> ()  [unwired: 1 in, 1 out]
            n137 = call <vilib>:"Add State(s) to Queue__jki_lib_state_machine.vi"("State(s) in Front (\"\")"="UI: Save Current State", "State(s) in (\"\")"=w286) -> ("States Out"=w285:string)  [unwired: 13 in]
          }
          event #3 {
            # "Discard the event because we'll close the front panel ourselves in Macro: Exit"
            # "Close Panel button (pressed) Event\n(this executes Macro: Exit to terminate the VI)"
            n138 = event-data() -> ()  [unwired: 1 in, 1 out]
            n139 = event-data("Discard?"=TRUE) -> ()  [unwired: 1 in, 1 out]
            n140 = call <vilib>:"Add State(s) to Queue__jki_lib_state_machine.vi"("State(s) in Front (\"\")"="Exit", "State(s) in (\"\")"=w292) -> ("States Out"=w291:string)  [unwired: 13 in]
          }
        }
      }
      frame #1 {
        # "Do not put any code in this frame.\n(it is a separator no-op)"
        n141 = call <vilib>:"Add State(s) to Queue__jki_lib_state_machine.vi"("State(s) in (\"\")"=w296) -> ("States Out"=w295:string)  [unwired: 14 in]
      }
      frame #2 {
        w306 = 42 items=["No error", "Argument error", "Memory is full", "Out of zone", "End of file", "File already open", "Generic file I/O error", "File not found", "File permission error", "Disk is full", "Duplicate path", "Too many files open", "System feature not enabled", "Resource file not found", "Cannot add resource", "Resource not found", "Image not found", "Image memory error", "Pen does not exist", "Config type invalid", "Config token not found", "Config parse error", "Config memory error", "Bad external code format", "Bad external code offset", "External code not present", "Null window", "Destroy window error", "Null menu", "Print aborted", "Bad print record", "Print driver error", "Windows error during printing", "Memory error during printing", "Print dialog error", "Generic print error", "Invalid device refnum", "Device not found", "Device parameter error", "Device unit error", "Cannot open device", "Device call aborted", "Generic error", "Cancelled by user", "Object ID too low", "Object ID too high", "Object not in heap", "Unknown heap", "Unknown object (invalid DefProc)", "Unknown object (DefProc not in table)", "Message out of range", "Invalid (null) method", "Unknown message", "Manager call not supported", "Bad address", "Network operation in progress", "Network operation timed out", "Connection is busy", "Network attribute not supported", "Network error", "Address in use", "System out of memory", "Connection aborted", "Connection refused", "Not connected", "Already connected", "Connection closed", "Initialization error (interapplication manager)", "Bad occurrence", "Wait on unbound occurrence handler", "Occurrence queue overflow", "Datalog type conflict", "Unused", "Unrecognized type (interapplication manager)", "Memory corrupt", "Failed to make temporary DLL", "Old CIN version", "Drag socket not found", "Failed to load drop-object", "Failed to register OLE object", "Failed to release OLE object", "Format specifier type mismatch", "Unknown format specifier", "Too few format specifiers", "Too many format specifiers", "Scan failed", "Newer CIN version", "Error converting to variant", "Runtime menu error", "Password tampered", "Variant attribute not found", "Incompatible variant data type", "Event data is not available", "Event Store is not present", "Occurrence is not found", "Event Queue is not created", "Event info is not available", "Refnum passed is NULL", "Error retrieving Class GUID", "Error retrieving CoClass GUID", "Error retrieving TypeLib GUID.", "Bad built application magic bytes.", "Specific driver is different from the specific driver associated with the Logical Name.", "There is no session opened to the class driver.", "Max Error", "MAX - Error with config objects", "MAX - Error loading configuration", "MAX - Group not supported"]
        # "Current State"
        # "Do not delete, rename, or modify this frame.\n(this is used to capture unhandled states and typos)"
        # "Handle mistyped state name (developer tool)"
        n142 = Format Into String(format string="Software Exception: Unhandled State \"%s\"." ("message"), error in=w302, w297) -> (resulting string=w305:string, error out=w304:errorcluster)  [unwired: 1 in]
        n143 = call <vilib>:"Error Cluster From Error Code.vi"("show call chain? (False)"=TRUE, "error in (no error)"=w304, "error message (\"\")"=w305, "error code (0)"=w306) -> ("error out"=w303:errorcluster)  [unwired: 5 in]
        n144 = call <vilib>:"Add State(s) to Queue__jki_lib_state_machine.vi"("State(s) in (\"\")"=w301) -> ("States Out"=w300:string)  [unwired: 14 in]
      }
      frame #3 {
        # "Do not delete, rename, or modify this frame.\n(this is used to determine panel behavior on exit)"
        # "originally closed?"
        # "exe?"
        # "If panel starts closed or is an EXE, then close it when we exit"
        n145 = property class="VI"() -> ("Front Panel.Open"=w315:bool)  [unwired: 2 in, 2 out]
        n146 = property class="App"() -> ("App.Kind"=w314:T13)  [unwired: 2 in, 2 out]
        n147 = control-ref of="Current VI Reference"() -> (w308:refnum<vi>)
        n148 = Not(x=w315) -> (.not. x?=w312:bool)
        n149 = Equal?(x=w314, y=T13."Run Time System" ("Application:Kind")) -> (x = y?=w311:bool)
        n150 = Or(x=w312, y=w311) -> (x .or. y?=w309:bool)
        n151 = Bundle By Name(cluster=w310, "Core.Current VI Reference"=w308, "Core.Close Panel on Exit?"=w309) -> (w317:T16)
        n152 = call <vilib>:"Add State(s) to Queue__jki_lib_state_machine.vi"("State(s) in (\"\")"=w319) -> ("States Out"=w318:string)  [unwired: 14 in]
      }
      frame #4 {
        # "Cleanup any data and references, here.\n(this is called automatically, by the Macro: Exit)"
        n153 = Unbundle By Name(w330) -> ("Core.Current VI Reference"=w333:refnum<vi>)
        n154 = Close Reference(reference=w333, error in (no error)=w332) -> (error out=w331:errorcluster)
        n155 = local read "1"() -> (w323:T1)
        n156 = local read "Agilent"() -> (w325:T1)
        n157 = local read "3"() -> (w320:T1)
        n158 = call <vilib>:"Release Semaphore Reference.vi"("semaphore"=w323) -> ("error out"=w329:errorcluster)  [unwired: 9 in, 1 out]
        n159 = call <vilib>:"Release Semaphore Reference.vi"("semaphore"=w320) -> ("error out"=w327:errorcluster)  [unwired: 9 in, 1 out]
        n160 = call <vilib>:"Release Semaphore Reference.vi"("error in (no error)"=w329, "semaphore"=w325) -> ("error out"=w326:errorcluster)  [unwired: 8 in, 1 out]
        n161 = local read "2"() -> (w321:T1)
        n162 = local read "4"() -> (w324:T1)
        n163 = call <vilib>:"Release Semaphore Reference.vi"("error in (no error)"=w327, "semaphore"=w321) -> ("error out"=w328:errorcluster)  [unwired: 8 in, 1 out]
        n164 = call <vilib>:"Release Semaphore Reference.vi"("error in (no error)"=w326, "semaphore"=w324) -> ()  [unwired: 8 in, 2 out]
        n165 = local read "1A"() -> (w322:T1)
        n166 = call <vilib>:"Release Semaphore Reference.vi"("error in (no error)"=w328, "semaphore"=w322) -> ()  [unwired: 8 in, 2 out]
        n167 = call <vilib>:"Add State(s) to Queue__jki_lib_state_machine.vi"("State(s) in (\"\")"=w335) -> ("States Out"=w334:string)  [unwired: 14 in]
      }
      frame #5 {
        # "Handle any errors here.\nYou can also output any states to clean-up after errors occur"
        # "Clear error"
        n168 = local read "Debug"() -> (w336:bool)
        n169 = case shown="True" w336 {
          tunnel: w337 -> [_ w349]
          frame #0 {
          }
          frame #1 {
            # "Unhandled Error -- Display it"
            n170 = call <vilib>:"General Error Handler.vi"("error in (no error)"=w349) -> ()  [unwired: 10 in, 5 out]
          }
        }
        n171 = Unbundle By Name(w337) -> ("source"=w341:string)
        n172 = local read "Control Error List"() -> (w343:string)
        n173 = Concatenate Strings("Error CONT: " ("string"), w341) -> (w339:string)
        n174 = local write "User Message"(w339) -> ()
        n175 = Concatenate Strings(w341, "\n", w343) -> (→"Control Error List":string)
        n176 = call <vilib>:"Add State(s) to Queue__jki_lib_state_machine.vi"("State(s) in Front (\"\")"="/* Post Error States", "State(s) in (\"\")"=w348) -> ("States Out"=w347:string)  [unwired: 13 in]
      }
      frame #6 {
        # "Do not put any code in this frame.\n(No errors that occur here will be handled.)"
        n177 = local read "All Agilent Refs"() -> (w350:refnum<visa-resource-name>[])
        n178 = for {
          tunnel: w350 -> [w356] mode=indexing
          n179 = VISA Close(VISA resource name=w356) -> ()  [unwired: 1 in, 1 out]
        }
        n180 = call <vilib>:"Add State(s) to Queue__jki_lib_state_machine.vi"("State(s) in (\"\")"=w355) -> ("States Out"=w354:string)  [unwired: 14 in]
      }
      frame #7 {
        # "Do not put any code in this frame.\n(It is a separator no-op. You can make a copy of this frame to create a new Data frame)"
        n181 = call <vilib>:"Add State(s) to Queue__jki_lib_state_machine.vi"("State(s) in (\"\")"=w360) -> ("States Out"=w359:string)  [unwired: 14 in]
      }
      frame #8 {
        w369 = refnum<visa-resource-name>[] ["AGILENT1", "AGILENT2", "AGILENT3", "AGILENT4", "AGILENT5", "AGILENT6"]  # Agilent Refs
        w370 = T17 {"Current VI Reference"=refnum, "Close Panel on Exit?"=FALSE}  # Core
        # "Data names and types of shift register data are defined by this bundle."
        # "Initialize the shift-register data, here.\n(data names are defined by what you wire into the bundle function)"
        n182 = Bundle("Core"=w370, "Agilent Refs"=w369, "GUI Aisle Top"="GUI Aisle Top", "GUI Aisle Mid"="GUI Aisle Mid", "GUI Aisle Bot"="GUI Aisle Bot", "Station Timer"="Station Timer", "Station Test State"="Station Test State", "Saved Test State"="Saved Test State", "Dryer Bank Filename"="Dryer Bank Filename", "Station Com List"="Station Com List") -> (w372:T16)  [unwired: 1 in]
        n183 = call <vilib>:"Add State(s) to Queue__jki_lib_state_machine.vi"("State(s) in (\"\")"=w374) -> ("States Out"=w373:string)  [unwired: 14 in]
        "All Agilent Refs" <- w369
      }
      frame #9 {
        w403 = Update_Wilt_GUI_Control."Init Station Number" ("Enum")
        # "Initialization Macro\n(This is called once, when the VI starts)"
        n184 = global read "Globals HCC.vi" "Label Com Array"() -> (w395:string[][])
        n185 = Transpose 2D Array(2D array=w395) -> (transposed array=w399:string[][])
        n186 = Transpose 2D Array(2D array=w395) -> (transposed array=w396:string[][])
        n187 = call "Array-Get 1D Row fr 2D str.vi"("all rows"=w399, "row index"=0) -> ("row"=w394:string[])  [unwired: 13 in]
        n188 = call "Array-Get 1D Row fr 2D str.vi"("all rows"=w396, "row index"=1) -> ("row"=w389:string[])  [unwired: 13 in]
        n189 = Decimal String To Number(string=w389, default (0L)=u8 0 ("default (0 I32)")) -> (number=w382:u8[])  [unwired: 1 in, 1 out]
        n190 = Delete From Array(array=w394, length=10, index=0) -> (deleted portion=w388:string[], array with subset deleted=w385:string[])
        n191 = Delete From Array(array=w382, length=10, index=0) -> (deleted portion=w377:u8[], array with subset deleted=w378:u8[])
        n192 = Delete From Array(array=w385, length=10, index=0) -> (deleted portion=w384:string[], array with subset deleted=w383:string[])
        n193 = Delete From Array(array=w378, length=10, index=0) -> (deleted portion=w376:u8[], array with subset deleted=w375:u8[])
        n194 = local read "GUI Aisle Top"() -> (w402:T4[])
        n195 = local read "GUI Aisle Bot"() -> (w400:T4[])
        n196 = local read "GUI Aisle Mid"() -> (w401:T4[])
        n197 = for {
          tunnel: w402 -> [_] mode=indexing
          tunnel: w377 -> [w419] mode=indexing
          tunnel: [w422] -> w404 mode=indexing
          tunnel: w403 -> [w421]
          tunnel: w388 -> [w420] mode=indexing
          n198 = call "Washer HCC GUI.vi"("Enum"=w421, "Station Number In"=w420, "Com Port In"=w419) -> ("Washer Out"=w422:T4)  [unwired: 10 in, 2 out]
        }
        n199 = for {
          tunnel: w401 -> [_] mode=indexing
          tunnel: w376 -> [w415] mode=indexing
          tunnel: [w418] -> w405 mode=indexing
          tunnel: w403 -> [w417]
          tunnel: w384 -> [w416] mode=indexing
          n200 = call "Washer HCC GUI.vi"("Enum"=w417, "Station Number In"=w416, "Com Port In"=w415) -> ("Washer Out"=w418:T4)  [unwired: 10 in, 2 out]
        }
        n201 = for {
          tunnel: w400 -> [_] mode=indexing
          tunnel: w375 -> [w411] mode=indexing
          tunnel: [w414] -> w406 mode=indexing
          tunnel: w403 -> [w413]
          tunnel: w383 -> [w412] mode=indexing
          n202 = call "Washer HCC GUI.vi"("Enum"=w413, "Station Number In"=w412, "Com Port In"=w411) -> ("Washer Out"=w414:T4)  [unwired: 10 in, 2 out]
        }
        n203 = local write "GUI Aisle Top"(w404) -> ()
        n204 = local write "GUI Aisle Mid"(w405) -> ()
        n205 = local write "GUI Aisle Bot"(w406) -> ()
        n206 = call <vilib>:"Add State(s) to Queue__jki_lib_state_machine.vi"("State(s) in (\"\")"=w410) -> ("States Out"=w409:string)  [unwired: 14 in]
      }
      frame #10 {
        # "If State is Wait Com, set timer for first broadcast."
        # "Initialization Macro\n(This is called once, when the VI starts)"
        n207 = local read "GUI Aisle Top"() -> (w429:T4[])
        n208 = local read "GUI Aisle Bot"() -> (w431:T4[])
        n209 = local read "GUI Aisle Mid"() -> (w430:T4[])
        n210 = Build Array (concatenate)(w431, w430, w429) -> (w426:T4[])
        n211 = for {
          tunnel: w426 -> [w445] mode=indexing
          tunnel: [w440] -> w424 mode=indexing
          tunnel: [w436] -> w425 mode=indexing
          tunnel: [w435] -> w423 mode=indexing
          n212 = Unbundle By Name(w445) -> ("Serial Number"=w444:string, "Com Port"=w435:u8)
          n213 = call "E-Time.vi"() -> ("Elapsed Time (sec)"=w437:dbl)  [unwired: 9 in, 2 out]
          n214 = Equal?(x=w444, y="") -> (x = y?=w439:bool)
          n215 = Select(t=Dryer_Test_State."No SN" ("Test State"), s=w439, f=Dryer_Test_State."Wait Com" ("Test State")) -> (s? t:f=w440:T10)
          n216 = Select(t=0.0, s=w439, f=w437) -> (s? t:f=w436:dbl)
        }
        n217 = local write "Station Com List"(w423) -> ()
        n218 = Bundle By Name(cluster=w428, "Saved Test State"=w424, "Station Test State"=w424, "Station Timer"=w425, "Station Com List"=w423) -> (w427:T16)
        n219 = call <vilib>:"Add State(s) to Queue__jki_lib_state_machine.vi"("State(s) in (\"\")"=w434) -> ("States Out"=w433:string)  [unwired: 14 in]
      }
      frame #11 {
        # "SKIP!"
        n220 = Unbundle By Name(w456) -> ("Agilent Refs"=w452:refnum<visa-resource-name>[])
        n221 = call "Agilent Channels.vi"("file path (dialog if empty)"="Agilent Channel Assignment") -> ("Station Data Headers"=→"Agilent Station Data Headers":string[][], "Index Array"=→"Agilent Station Data Index Array":i32[][], "Agilent Channels To Read"=w450:T9[], "Agilent Channel Water Valves"=→"Agilent Channels Water Valves":T9[])  [unwired: 10 in, 1 out]
        "Agilent Read Channels Array" <- w450
        n222 = for {
          tunnel: [w469] -> w457
          tunnel: w452 -> [w462] mode=indexing
          tunnel: w455 -> [w468]
          tunnel: w450 -> [w465]
          shift-right: [w463] -> w448
          shift-left: refnum<visa-resource-name>[] [] -> [w461]
          i -> [w467]
          n223 = Increment(x=w467) -> (x+1=w466:i32)
          n224 = call "Init Agilent Channels Wilt.vi"("Agilent Number"=w466, "VISA Resource Name"=w462, "Agilent Channels Array"=w465, "error in (no error)"=w468) -> ("Number of Read Channels"=w464:i32, "error out"=w469:errorcluster)  [unwired: 10 in]
          n225 = Greater Than 0?(x=w464) -> (x > 0?=w460:bool)
          n226 = case shown="True" w460 {
            tunnel: [w470 w473] -> w463
            tunnel: w462 -> [_ w472]
            tunnel: w461 -> [w470 w471]
            frame #0 {
            }
            frame #1 {
              n227 = Build Array (concatenate)(w471, w472) -> (w473:refnum<visa-resource-name>[])
            }
          }
        }
        "Agilent Read Refs" <- w448
        n228 = case shown="Error" w457 {
          selector: w457 -> [_ w476]
          tunnel: w451 -> [_ w477]
          frame #0 {
          }
          frame #1 {
            n229 = Unbundle By Name(w476) -> ("source"=w475:string)
            n230 = Concatenate Strings("Error: " ("string"), w477, w475) -> (w474:string)
            n231 = One Button Dialog(message=w474) -> ()  [unwired: 1 in, 1 out]
          }
        }
        n232 = call <vilib>:"Add State(s) to Queue__jki_lib_state_machine.vi"("State(s) in (\"\")"=w459) -> ("States Out"=w458:string)  [unwired: 14 in]
      }
      frame #12 {
        # "Fixme! once com [oprts in"
        # "Do not put any code in this frame.\nInitialize all the com ports to GEA2 specs."
        n233 = local read "All Confgured Com Array"() -> (w487:u8[])
        n234 = call "Find Valid Com Ports.vi"("Valid Com Port List(100,2:56)"=w487) -> ("Valid Com Ports"=w486:refnum<visa-resource-name>[])  [unwired: 13 in, 1 out]
        n235 = for {
          tunnel: w486 -> [w495] mode=indexing
          tunnel: [w495] -> _
          tunnel: w485 -> [w498]
          tunnel: [w496] -> w480
          shift-right: [w494] -> w483
          shift-left: u8[] [] ("All Com Array") -> [w493]
          tunnel: [w492] -> w482 mode=indexing
          n236 = call "GEA2_ICP_Washer_SM.vi"("ComPort"=w495, "Mode"=GEA2_Dryer_Interface_Ctrl."Init Com Port", "Error In"=w498) -> ("Dryer Status Serial Data Out"=w492:T2, "Error Out"=w496:errorcluster)  [unwired: 7 in, 4 out]
          n237 = case shown="No Error" w496 {
            tunnel: w495 -> [w501 w504]
            tunnel: [w500 w503] -> w494
            tunnel: w493 -> [w502 w503]
            frame #0 {
              n238 = call "Com Chan Type Conversion.vi"("Com Chan In"=w501) -> ("Com Channel #"=w499:u8)  [unwired: 12 in, 2 out]
              n239 = Build Array (concatenate)(w502, w499) -> (w500:u8[])
            }
            frame #1 {
              w507 = "COM Init Error.  "
              n240 = Type Cast(type=w507, x=w504) -> (*(type *) &x=w505:string)
              n241 = Concatenate Strings(w507, w505) -> (w506:string)
              n242 = One Button Dialog(message=w506) -> ()  [unwired: 1 in, 1 out]
            }
          }
        }
        n243 = local write "All Confgured Com Array"(w483) -> ()
        n244 = local write "Dryer Com Info"(w482) -> ()
        n245 = call <vilib>:"Clear Errors.vi"("error in (no error)"=w480) -> ("error out"=w481:errorcluster)  [unwired: 6 in]
        n246 = case shown="Error" w480 {
          tunnel: [_ "Exit" ("State(s) in Front (\"\")")] -> w479
          frame #0 {
          }
          frame #1 {
          }
        }
        n247 = call <vilib>:"Add State(s) to Queue__jki_lib_state_machine.vi"("State(s) in Front (\"\")"=w479, "State(s) in (\"\")"=w490) -> ("States Out"=w489:string)  [unwired: 13 in]
      }
      frame #13 {
        # "Do not put any code in this frame.\n(It is a separator no-op. You can make a copy of this frame to create a new UI frame)"
        n248 = call <vilib>:"Add State(s) to Queue__jki_lib_state_machine.vi"("State(s) in (\"\")"=w511) -> ("States Out"=w510:string)  [unwired: 14 in]
      }
      frame #14 {
        # "Initialize the User Interface, here.\n(this is called automatically, by the Macro: Init)"
        n249 = global read "Globals HCC.vi" "No Com Color"() -> (→"No Com":u32)
        n250 = global read "Globals HCC.vi" "Stopped Color"() -> (→"Stopped":u32)
        n251 = global read "Globals HCC.vi" "Running Color"() -> (→"Running":u32)
        n252 = global read "Globals HCC.vi" "Err Color"() -> (→"Fault":u32)
        n253 = call <vilib>:"Add State(s) to Queue__jki_lib_state_machine.vi"("State(s) in (\"\")"=w519) -> ("States Out"=w518:string)  [unwired: 14 in]
      }
      frame #15 {
        # "Initialize the User Interface, here.\n(this is called automatically, by the Macro: Init)"
        n254 = flat-sequence {
          tunnel: [string[] ["Aisle1", "Aisle1A", "Aisle2", "Aisle3", "Aisle4"]] -> w523
          frame #0 {
            n255 = local write "User Message"("Saving Setup ") -> ()
          }
        }
        n256 = Unbundle By Name(w524) -> ("Dryer Bank Filename"=w522:path)
        n257 = for {
          tunnel: w523 -> [w536] mode=indexing
          tunnel: w522 -> [w534]
          shift-right: [w532] -> w520
          shift-left: w521 -> [w533]
          i -> [w537]
          n258 = case shown="0, Default" w537 {
            tunnel: [w538 w539 w540] -> w535
            frame #0 {
              n259 = local read "GUI Aisle Top"() -> (w538:T4[])
            }
            frame #1 {
              n260 = local read "GUI Aisle Mid"() -> (w539:T4[])
            }
            frame #2 {
              n261 = local read "GUI Aisle Bot"() -> (w540:T4[])
            }
          }
          n262 = call "File Washer HCC.vi"("Dryer Aisle In"=w535, "RW  Mode"=T11."Write Dryer Bank", "Dryer Bank Filename"=w534, "Aisle Label"=w536, "error in (no error)"=w533) -> ("error out"=w532:errorcluster)  [unwired: 7 in, 3 out]
        }
        n263 = flat-sequence {
          tunnel: w520 -> [_]
          frame #0 {
            n264 = local write "User Message"("") -> ()
            n265 = local write "Save Setup"(FALSE ("Save Setup")) -> ()
          }
        }
        n266 = call <vilib>:"Add State(s) to Queue__jki_lib_state_machine.vi"("State(s) in (\"\")"=w526) -> ("States Out"=w525:string)  [unwired: 14 in]
      }
      frame #16 {
        (unwired) T19."Read Dryer Bank" ("RW  Mode")
        # "Initialize the User Interface, here.\n(this is called automatically, by the Macro: Init)"
        n267 = Unbundle By Name(w545) -> ("Dryer Bank Filename"=w541:path)
        n268 = for {
          tunnel: string[] ["AisleTop", "Aisle Mid", "Aisle Bot", "Aisle3", "Aisle4"] -> [w555] mode=indexing
          shift-right: [w552] -> w542
          shift-left: w543 -> [w553]
          tunnel: w541 -> [w548]
          i -> [w551]
          n269 = case shown="2" w551 {
            tunnel: [w559 w560 w561] -> w554
            frame #0 {
              n270 = local read "GUI Aisle Top"() -> (w559:T4[])
            }
            frame #1 {
              n271 = local read "GUI Aisle Mid"() -> (w560:T4[])
            }
            frame #2 {
              n272 = local read "GUI Aisle Bot"() -> (w561:T4[])
            }
          }
          n273 = call "File Washer HCC.vi"("Dryer Aisle In"=w554, "RW  Mode"=T11."Read Dryer Bank", "Dryer Bank Filename"=w548, "Aisle Label"=w555, "error in (no error)"=w553) -> ("Dryer Aisle Out"=w550:T4[], "error out"=w552:errorcluster)  [unwired: 7 in, 2 out]
          n274 = case shown="2" w551 {
            tunnel: w550 -> [w556 w557 w558]
            frame #0 {
              n275 = local write "GUI Aisle Top"(w556) -> ()
            }
            frame #1 {
              n276 = local write "GUI Aisle Mid"(w557) -> ()
            }
            frame #2 {
              n277 = local write "GUI Aisle Bot"(w558) -> ()
            }
          }
        }
        n278 = call <vilib>:"Add State(s) to Queue__jki_lib_state_machine.vi"("State(s) in (\"\")"=w547) -> ("States Out"=w546:string)  [unwired: 14 in]
      }
      frame #17 {
        # "Argument"
        # "Set and Unset Cursor Busy.\n(Usage: \"UI: Cursor Set >> Busy|Idle\")"
        n279 = case shown="\"Idle\", Default" w562 {
          tunnel: w564 -> [w569 w571]
          tunnel: [w568 w570] -> w563
          frame #0 {
            n280 = call <vilib>:"Unset Busy.vi"("error in (no error)"=w569) -> ("error out"=w568:errorcluster)  [unwired: 10 in]
          }
          frame #1 {
            n281 = call <vilib>:"Set Busy.vi"("error in (no error)"=w571) -> ("error out"=w570:errorcluster)  [unwired: 9 in, 1 out]
          }
        }
        n282 = call <vilib>:"Add State(s) to Queue__jki_lib_state_machine.vi"("State(s) in (\"\")"=w567) -> ("States Out"=w566:string)  [unwired: 14 in]
      }
      frame #18 {
        # "Argument"
        # "Set Front Panel Open or Closed\n(Usage: \"UI: Front Panel State >> Open|Close\")"
        n283 = Unbundle By Name(w574) -> ("Core.Current VI Reference"=w573:refnum<vi>)
        n284 = case shown="\"Open\", Default" w572 {
          tunnel: w576 -> [w582 w595]
          tunnel: [w584 w596] -> w575
          tunnel: w573 -> [w583 w593]
          frame #0 {
            n285 = property class="VI"(reference=w583, error in=w582) -> (reference out=w580:refnum<vi>, error out=w581:errorcluster, "Front Panel.Open"=w579:bool)
            n286 = case shown="False" w579 {
              tunnel: [w587 w590] -> w584
              tunnel: w581 -> [w586 w590]
              tunnel: w580 -> [w585 _]
              frame #0 {
                n287 = invoke class="VI" method="FP.Open"(reference=w585, error in=w586, "Activate"=TRUE, "State"=T15."Standard") -> (error out=w587:errorcluster)  [unwired: 1 in, 4 out]
              }
              frame #1 {
              }
            }
          }
          frame #1 {
            n288 = property class="VI"(reference=w593, error in=w595) -> (reference out=w592:refnum<vi>, error out=w594:errorcluster, "Front Panel.Open"=w591:bool)
            n289 = case shown="True" w591 {
              tunnel: [w597 w600] -> w596
              tunnel: w594 -> [w597 w599]
              tunnel: w592 -> [_ w598]
              frame #0 {
              }
              frame #1 {
                n290 = invoke class="VI" method="FP.Close"(reference=w598, error in=w599) -> (error out=w600:errorcluster)  [unwired: 1 in, 2 out]
              }
            }
          }
        }
        n291 = call <vilib>:"Add State(s) to Queue__jki_lib_state_machine.vi"("State(s) in (\"\")"=w578) -> ("States Out"=w577:string)  [unwired: 14 in]
      }
      frame #19 {
        # "Do not put any code in this frame.\n(It is a separator no-op. You can make a copy of this frame to create a new Macro frame)"
        n292 = call <vilib>:"Add State(s) to Queue__jki_lib_state_machine.vi"("State(s) in (\"\")"=w604) -> ("States Out"=w603:string)  [unwired: 14 in]
      }
      frame #20 {
        # "Initialization Macro\n(This is called once, when the VI starts)"
        n293 = call <vilib>:"Add State(s) to Queue__jki_lib_state_machine.vi"("State(s) in (\"\")"=w608) -> ("States Out"=w607:string)  [unwired: 14 in]
      }
      frame #21 {
        # "Exit Macro\n(This is called once, when the VI exits)"
        n294 = Unbundle By Name(w615) -> ("Core.Close Panel on Exit?"=w614:bool)
        n295 = Select(t="UI: Front Panel State >> Close", s=w614, f="") -> (s? t:f=w611:string)
        n296 = call <vilib>:"Add State(s) to Queue__jki_lib_state_machine.vi"("State(s) in (\"\")"=w611, "State(s) at Back (\"\")"="Data: Cleanup\nExit") -> ("States Out"=w609:string)  [unwired: 13 in]
        n297 = call <vilib>:"Add State(s) to Queue__jki_lib_state_machine.vi"("State(s) in Front (\"\")"=w609, "State(s) in (\"\")"=w618) -> ("States Out"=w617:string)  [unwired: 13 in]
      }
      frame #22 {
        # "Start Datalogging and Start Test.  Datalogging continues on its own loop.\nUpdating the gui and saving data is a second loop.\n\nThe test will continue."
        # "Template Separator\n(You can make a copy of, or modify, this frame)"
        n298 = call <vilib>:"Add State(s) to Queue__jki_lib_state_machine.vi"("State(s) in (\"\")"=w622) -> ("States Out"=w621:string)  [unwired: 14 in]
      }
      frame #23 {
        # "Your code here.\n(You can make a copy of, or modify, this frame)"
        n299 = flat-sequence {
          frame #0 {
            w627 = TRUE ("Init Complete")
            n300 = property on="Init Complete" class="Bool (strict)"("Val(Sgnl)"=w627) -> ()  [unwired: 2 in, 2 out]
            "Init Complete" <- w627
          }
        }
        n301 = call <vilib>:"Add State(s) to Queue__jki_lib_state_machine.vi"("State(s) in (\"\")"=w626) -> ("States Out"=w625:string)  [unwired: 14 in]
      }
      frame #24 {
        # "Template Separator\n(You can make a copy of, or modify, this frame)"
        n302 = call <vilib>:"Add State(s) to Queue__jki_lib_state_machine.vi"("State(s) in (\"\")"=w631) -> ("States Out"=w630:string)  [unwired: 14 in]
      }
      frame #25 {
        # "Wait for end."
        # "Your code here.\n(You can make a copy of, or modify, this frame)"
        n303 = local read "GUI Aisle Top"() -> (w633:T4[])
        n304 = local read "GUI Aisle Bot"() -> (w635:T4[])
        n305 = local read "GUI Aisle Mid"() -> (w634:T4[])
        n306 = Build Array (concatenate)(w635, w634, w633) -> (→"All Test Stations":T4[])
        n307 = call <vilib>:"Add State(s) to Queue__jki_lib_state_machine.vi"("State(s) in (\"\")"=w639) -> ("States Out"=w638:string)  [unwired: 14 in]
      }
      frame #26 {
        # "Ifserial number is changed from \"\" to something, then state goes to Wait Com.  This implies that\nthe user should change the serial number before installing a new dryer."
        n308 = Unbundle By Name(w644) -> ("Station Test State"=w641:T10[])
        n309 = local read "All Test Stations"() -> (w645:T4[])
        n310 = for {
          tunnel: w645 -> [w657] mode=indexing
          tunnel: [w650] -> w642 mode=indexing
          tunnel: w641 -> [w649] mode=indexing
          n311 = Unbundle By Name(w657) -> ("Serial Number"=w656:string)
          n312 = Not Equal?(x=w656, y="") -> (x != y?=w652:bool)
          n313 = Equal?(x=w649, y=Dryer_Test_State."No SN" ("Test State")) -> (x = y?=w653:bool)
          n314 = And(x=w652, y=w653) -> (x .and. y?=w651:bool)
          n315 = Select(t=Dryer_Test_State."Wait Com" ("Test State"), s=w651, f=w649) -> (s? t:f=w650:T10)
        }
        n316 = Bundle By Name(cluster=w644, "Station Test State"=w642) -> (w643:T16)
        n317 = call <vilib>:"Add State(s) to Queue__jki_lib_state_machine.vi"("State(s) in (\"\")"=w647) -> ("States Out"=w646:string)  [unwired: 14 in]
      }
      frame #27 {
        # "Note the or is for dryer simulation, since the laptops can't ack in time.  Assume that some bytes there means that it has received the message."
        # "Do not put any code in this frame.\nInitialize all the com ports to GEA2 specs."
        n318 = Unbundle By Name(w665) -> ("Station Timer"=w671:dbl[], "Station Test State"=w659:T10[], "Station Com List"=w661:u8[])
        n319 = call "E-Time.vi"() -> ("Elapsed Time (sec)"=w674:dbl)  [unwired: 9 in, 2 out]
        n320 = local write "Station Test State"(w659) -> ()
        n321 = local read "All Confgured Com Array"() -> (w663:u8[])
        n322 = Subtract(x=w674, y=w671) -> (x-y=w673:dbl[])
        n323 = Subtract(x=w673, y="Wait Com Timer") -> (x-y=w670:dbl[])
        n324 = Equal?(x=w659, y=Dryer_Test_State."Wait Com" ("Test State")) -> (x = y?=w669:bool[])
        n325 = Greater Than 0?(x=w670) -> (x > 0?=w668:bool[])
        n326 = And(x=w668, y=w669) -> (x .and. y?=w667:bool[])
        n327 = for {
          tunnel: w671 -> [w693]
          tunnel: w667 -> [w700]
          tunnel: [w694] -> w666
          tunnel: w663 -> [w695] mode=indexing
          tunnel: w676 -> [w701]
          tunnel: [w690] -> w660
          tunnel: w661 -> [w696]
          shift-right: [w687] -> w658
          shift-left: w659 -> [w689]
          n328 = Search 1D Array(1D array=w696, element=w695) -> (index of element=w688:i32)  [unwired: 1 in]
          n329 = Index Array(array=w700, index=w688) -> (element=w697:bool)
          n330 = Index Array(array=w693, index=w688) -> (element=w698:dbl)
          n331 = case shown="True" w697 {
            tunnel: w701 -> [w711 w725]
            tunnel: [w711 w716] -> w691
            tunnel: [_ w715] -> w699
            tunnel: [w710 w723] -> w692
            tunnel: w698 -> [w710 _]
            tunnel: w695 -> [_ w722]
            tunnel: [w709 w720] -> w687
            tunnel: w689 -> [w709 w721]
            tunnel: w688 -> [_ w719]
            frame #0 {
            }
            frame #1 {
              n332 = call "Com Chan Type Conversion.vi"("Com Chan"=w722) -> ("VISA resource name"=w715:refnum<visa-resource-name>)  [unwired: 12 in, 2 out]
              n333 = call "GEA2_ICP_Washer_SM.vi"("ComPort"=w715, "Mode"=GEA2_Dryer_Interface_Ctrl."Send WILT Startup CMDs", "Error In"=w725) -> ("WriteOK"=w717:bool, "Error Out"=w716:errorcluster)  [unwired: 7 in, 4 out]
              n334 = property class="Instr"(reference=w715, error in=w716) -> ("Serial Settings:Number of Bytes at Serial Port"=w714:u32)  [unwired: 2 out]
              "WC Bytes" <- w714
              n335 = Greater Than 0?(x=w714) -> (x > 0?=w712:bool)
              "WC x > 0?" <- w712
              n336 = Or(x=w712, y=w717) -> (x .or. y?=w713:bool)
              n337 = case shown="True" w713 {
                tunnel: [Dryer_Test_State."Wait Com" ("Test State") Dryer_Test_State."Wait to Start" ("Test State")] -> w718
                frame #0 {
                }
                frame #1 {
                }
              }
              n338 = Replace Array Subset(array=w721, new element=w718, index=w719) -> (w720:T10[])
              n339 = call "E-Time.vi"() -> ("Elapsed Time (sec)"=w723:dbl)  [unwired: 9 in, 2 out]
            }
          }
          n340 = case shown="Error" w691 {
            selector: w691 -> [w702 w705]
            tunnel: w699 -> [_ w706]
            tunnel: [w702 w704] -> w690
            frame #0 {
            }
            frame #1 {
              w708 = "Wait COM Error.  "
              n341 = Type Cast(type=w708, x=w706) -> (*(type *) &x=w707:string)
              n342 = Concatenate Strings(w708, w707) -> (w703:string)
              n343 = call <vilib>:"Clear Errors.vi"("error in (no error)"=w705) -> ("error out"=w704:errorcluster)  [unwired: 6 in]
              n344 = local write "User Message"(w703) -> ()
            }
          }
          n345 = Replace Array Subset(array=w693, new element=w692, index=w688) -> (w694:dbl[])
        }
        n346 = stacked-sequence {
          tunnel: [w680] -> w662
          tunnel: w660 -> [_]
          frame #0 {
            n347 = local read "Save Setup"() -> (w679:bool)
            n348 = local read "Stop Test"() -> (w681:bool)
            n349 = case shown="False" w681 {
              tunnel: [w683 "UI: Save Current State\nExit" ("State(s) in Front (\"\")")] -> w680
              tunnel: w679 -> [w682 _]
              frame #0 {
                n350 = case shown="True" w682 {
                  tunnel: ["Check Wait" ("State(s) in Front (\"\")") "UI: Save Current State\nCheck Wait" ("State(s) in Front (\"\")")] -> w683
                  frame #0 {
                  }
                  frame #1 {
                  }
                }
              }
              frame #1 {
              }
            }
          }
        }
        n351 = Bundle By Name(cluster=w665, "Station Timer"=w666, "Station Test State"=w658) -> (w664:T16)
        n352 = call <vilib>:"Add State(s) to Queue__jki_lib_state_machine.vi"("State(s) in Front (\"\")"=w662, "State(s) in (\"\")"=w678) -> ("States Out"=w677:string)  [unwired: 13 in]
      }
      frame #28 {
        # "Wait for both status and log to be reported."
        n353 = Unbundle By Name(w736) -> ("Station Test State"=w728:T10[], "Station Timer"=w730:dbl[])
        n354 = local read "All Test Stations"() -> (w732:T4[])
        n355 = local write "Station Test State"(w728) -> ()
        n356 = Equal?(x=w728, y=Dryer_Test_State."Wait to Start" ("Test State")) -> (x = y?=w733:bool[])
        n357 = disable-structure shown="Enabled" {
          disable-tunnel: w733 -> [w745 _]
          disable-tunnel: w732 -> [w744 _]
          disable-tunnel: [w743 w773] -> w731
          disable-tunnel: w730 -> [w742 w772]
          disable-tunnel: [w741 w772] -> w729
          disable-tunnel: w728 -> [w740 w773]
          frame #0 {
            # "The check is that both string lengths are > 0. Assumes that these are initializied to \"\".\nReset the timer value to the current time once you wait to start."
            n358 = for {
              tunnel: w745 -> [w751] mode=indexing
              tunnel: w744 -> [w750] mode=indexing
              tunnel: [w749] -> w743 mode=indexing
              tunnel: w740 -> [w748] mode=indexing
              tunnel: w742 -> [w747] mode=indexing
              tunnel: [w746] -> w741 mode=indexing
              i -> [w752]
              n359 = case shown="True" w751 {
                tunnel: w752 -> [_ _]
                tunnel: w750 -> [_ w769]
                tunnel: [w754 w760] -> w749
                tunnel: w748 -> [w754 _]
                tunnel: w747 -> [w753 w757]
                tunnel: [w753 w759] -> w746
                frame #0 {
                }
                frame #1 {
                  n360 = Unbundle By Name(w769) -> ("Sample Record(t, CC, ASCII, Status )"=w768:string[])
                  n361 = Index Array(array=w768, index #1=3 ("disabled index (col)"), index #2=4 ("disabled index (col)")) -> (element #1=w767:string, element #2=w766:string)
                  n362 = String Length(string=w767) -> (length=w765:i32)
                  n363 = String Length(string=w766) -> (length=w764:i32)
                  n364 = Multiply(x=w765, y=w764) -> (x*y=w763:i32)
                  n365 = Not Equal To 0?(x=w763) -> (x != 0?=w758:bool)
                  n366 = case shown="True" w758 {
                    tunnel: [w770 w771] -> w759
                    tunnel: w757 -> [w770 _]
                    frame #0 {
                    }
                    frame #1 {
                      n367 = call "E-Time.vi"() -> ("Elapsed Time (sec)"=w771:dbl)  [unwired: 9 in, 2 out]
                    }
                  }
                  n368 = Select(t=Dryer_Test_State."Wait to Start" ("Test State"), s=w758, f=Dryer_Test_State."Wait Com" ("Test State")) -> (s? t:f=w760:T10)
                }
              }
            }
          }
          frame #1 {
            # "Not sure why this is here, to verify the output of wait com.\nThis depends on the periodic output of the serial port.  It is not \nlike this in the  first real dryer."
          }
        }
        n369 = Bundle By Name(cluster=w736, "Station Test State"=w731, "Station Timer"=w729) -> (w735:T16)
        n370 = call <vilib>:"Add State(s) to Queue__jki_lib_state_machine.vi"("State(s) in (\"\")"=w739) -> ("States Out"=w738:string)  [unwired: 14 in]
      }
      frame #29 {
        # "If the color is indicating fault, set test state to fault.  Reset will reset back to Wait Com.\nA notice will be sent to user notice block in the case of a fault."
        n371 = Unbundle By Name(w778) -> ("Station Test State"=w777:T10[])
        n372 = global read "Globals HCC.vi" "Fault Color"() -> (w774:u32)
        n373 = local read "All Test Stations"() -> (w780:T4[])
        n374 = Equal?(x=w777, y=Dryer_Test_State."Temp Fault" ("Test State")) -> (x = y?=w781:bool[])
        n375 = for {
          tunnel: w781 -> [w795] mode=indexing
          tunnel: w780 -> [w794] mode=indexing
          tunnel: [w793] -> w779 mode=indexing
          tunnel: w777 -> [w792] mode=indexing
          tunnel: [w791] -> w776
          tunnel: "Reset Faults" -> [w790]
          tunnel: w774 -> [w789]
          n376 = case shown="False" w795 {
            tunnel: w794 -> [w804 _]
            tunnel: [w801 w810] -> w793
            tunnel: w792 -> [_ w809]
            tunnel: [w799 w808] -> w791
            tunnel: w790 -> [w799 w808]
            tunnel: w789 -> [w796 _]
            frame #0 {
              n377 = Unbundle By Name(w804) -> ("Station Number"=w797:string, "Status Color"=w800:u32)
              n378 = Equal?(x=w800, y=w796) -> (x = y?=w798:bool)
              n379 = Select(t=Dryer_Test_State."Temp Fault" ("Test State"), s=w798, f=Dryer_Test_State."Wait Com" ("Test State")) -> (s? t:f=w801:T10)
              n380 = case shown="True" w798 {
                tunnel: w797 -> [_ w805]
                frame #0 {
                }
                frame #1 {
                  n381 = Concatenate Strings("Temp Fault Station " ("string"), w805) -> (w807:string)
                  n382 = local write "User Message"(w807) -> ()
                }
              }
            }
            frame #1 {
              n383 = case shown="True" w808 {
                tunnel: [w811 Dryer_Test_State."Wait Com" ("Test State")] -> w810
                tunnel: w809 -> [w811 _]
                frame #0 {
                }
                frame #1 {
                }
              }
            }
          }
        }
        n384 = Bundle By Name(cluster=w778, "Station Test State"=w779) -> (w783:T16)
        n385 = case shown="True" w776 {
          frame #0 {
          }
          frame #1 {
            n386 = local write "User Message"("" ("User Notice")) -> ()
            n387 = local write "Reset Faults"(FALSE ("Reset Faults")) -> ()
          }
        }
        n388 = call <vilib>:"Add State(s) to Queue__jki_lib_state_machine.vi"("State(s) in (\"\")"=w786) -> ("States Out"=w785:string)  [unwired: 14 in]
      }
      frame #30 {
        # "The check is that both string lengths are > 0. Assumes that these are initializied to \"\""
        # "Wait for both status and log to be reported."
        n389 = Unbundle By Name(w819) -> ("Station Test State"=w813:T10[], "Station Timer"=w815:dbl[])
        n390 = local read "All Test Stations"() -> (w821:T4[])
        n391 = Equal?(x=Dryer_Test_State."Wait to Start" ("Test State"), y=w813) -> (x = y?=w822:bool[])
        n392 = local write "Station Test State"(w813) -> ()
        n393 = for {
          tunnel: w822 -> [w830] mode=indexing
          tunnel: w821 -> [w829] mode=indexing
          tunnel: [w828] -> w817 mode=indexing
          tunnel: w813 -> [w827] mode=indexing
          tunnel: w815 -> [w826] mode=indexing
          tunnel: [w825] -> w814 mode=indexing
          n394 = case shown="True" w830 {
            tunnel: w829 -> [_ w845]
            tunnel: [w832 w836] -> w828
            tunnel: w827 -> [w832 _]
            tunnel: w826 -> [w831 w833]
            tunnel: [w831 w835] -> w825
            frame #0 {
            }
            frame #1 {
              n395 = Unbundle By Name(w845) -> ("Dryer Details.Status"=w842:string)
              n396 = call "E-Time.vi"() -> ("Elapsed Time (sec)"=w841:dbl)  [unwired: 9 in, 2 out]
              n397 = Subtract(x=w841, y=w833) -> (x-y=w840:dbl)
              n398 = call "Type Conv - Dryer Status to Txt.vi"("Status"=Dryer_Status_Ctrl."Cycle Running") -> ("Ring Text.Text"=w843:string)  [unwired: 10 in]
              n399 = Subtract(x=w840, y="Resend Start Limit") -> (x-y=w838:dbl)
              n400 = Greater Than 0?(x=w838) -> (x > 0?=w834:bool)
              n401 = Equal?(x=w842, y=w843) -> (x = y?=w837:bool)
              n402 = case shown="False" w837 {
                tunnel: [w848 Dryer_Test_State."Watering" ("Test State")] -> w836
                tunnel: [w847 0.0 ("element")] -> w835
                tunnel: w834 -> [w849 _]
                tunnel: w833 -> [w846 _]
                frame #0 {
                  n403 = case shown="False" w849 {
                    tunnel: [Dryer_Test_State."Wait to Start" ("Test State") Dryer_Test_State."Wait Com" ("Test State")] -> w848
                    tunnel: [w850 w853] -> w847
                    tunnel: w846 -> [w850 w853]
                    frame #0 {
                      # "Wait"
                    }
                    frame #1 {
                      # "Resend Command"
                    }
                  }
                }
                frame #1 {
                  # "Continue.  Having a timer\nvalue of 0 is trigger to turn on valve"
                }
              }
            }
          }
        }
        n404 = Bundle By Name(cluster=w819, "Station Test State"=w817, "Station Timer"=w814) -> (w818:T16)
        n405 = call <vilib>:"Add State(s) to Queue__jki_lib_state_machine.vi"("State(s) in (\"\")"=w824) -> ("States Out"=w823:string)  [unwired: 14 in]
      }
      frame #31 {
        # "Keyword New, means dryer has been replaced during dry cycle"
        # "The check is that both string lengths are > 0. Assumes that these are initializied to \"\""
        # "Wait for both status and log to be reported."
        n406 = Unbundle By Name(w863) -> ("Station Test State"=w856:T10[], "Station Timer"=w857:dbl[])
        n407 = local read "All Test Stations"() -> (w864:T4[])
        n408 = Equal?(x=Dryer_Test_State."Drying" ("Test State"), y=w856) -> (x = y?=w865:bool[])
        n409 = local write "Station Test State"(w856) -> ()
        n410 = for {
          tunnel: w865 -> [w873] mode=indexing
          tunnel: w864 -> [w872] mode=indexing
          tunnel: [w871] -> w861 mode=indexing
          tunnel: w856 -> [w870] mode=indexing
          tunnel: [w869] -> w858 mode=indexing
          tunnel: w857 -> [w868] mode=indexing
          n411 = case shown="True" w873 {
            tunnel: w872 -> [_ w885]
            tunnel: [w875 w883] -> w871
            tunnel: w870 -> [w875 w882]
            tunnel: [w874 w881] -> w869
            tunnel: w868 -> [w874 w880]
            frame #0 {
            }
            frame #1 {
              n412 = Unbundle By Name(w885) -> ("Dryer Details.Status"=w879:string)
              n413 = Match Pattern(string=w879, regular expression="New") -> (offset past match=w877:i32)  [unwired: 1 in, 3 out]
              n414 = call "Type Conv - Dryer Status to Txt.vi"("Status"=Dryer_Status_Ctrl."Cycle Completed") -> ("Ring Text.Text"=w887:string)  [unwired: 10 in]
              n415 = Greater Or Equal To 0?(x=w877) -> (x >= 0?=w876:bool)
              n416 = Equal?(x=w879, y=w887) -> (x = y?=w884:bool)
              n417 = case shown="False" w884 {
                tunnel: [w889 Dryer_Test_State."Cooldown" ("Test State")] -> w883
                tunnel: w882 -> [w888 _]
                tunnel: [w891 w897] -> w881
                tunnel: w880 -> [w890 _]
                tunnel: w876 -> [w892 _]
                frame #0 {
                  n418 = case shown="True" w892 {
                    tunnel: [w894 w896] -> w891
                    tunnel: w890 -> [w894 w896]
                    tunnel: [w893 Dryer_Test_State."Wait Com" ("Test State")] -> w889
                    tunnel: w888 -> [w893 _]
                    frame #0 {
                    }
                    frame #1 {
                    }
                  }
                }
                frame #1 {
                  n419 = call "E-Time.vi"() -> ("Elapsed Time (sec)"=w897:dbl)  [unwired: 9 in, 2 out]
                }
              }
            }
          }
        }
        n420 = Bundle By Name(cluster=w863, "Station Test State"=w861, "Station Timer"=w858) -> (w862:T16)
        n421 = call <vilib>:"Add State(s) to Queue__jki_lib_state_machine.vi"("State(s) in (\"\")"=w867) -> ("States Out"=w866:string)  [unwired: 14 in]
      }
      frame #32 {
        # "The check is that both string lengths are > 0. Assumes that these are initializied to \"\""
        # "Wait for both status and log to be reported."
        n422 = Unbundle By Name(w908) -> ("Station Test State"=w901:T10[], "Station Timer"=w904:dbl[], "Station Com List"=w899:u8[])
        n423 = Equal?(x=Dryer_Test_State."Cooldown" ("Test State"), y=w901) -> (x = y?=w909:bool[])
        n424 = local write "Station Test State"(w901) -> ()
        n425 = for {
          tunnel: w909 -> [w918] mode=indexing
          tunnel: [w917] -> w906 mode=indexing
          tunnel: w901 -> [w916] mode=indexing
          tunnel: w904 -> [w915] mode=indexing
          tunnel: w903 -> [w914]
          tunnel: [w913] -> w902
          tunnel: w899 -> [w912] mode=indexing
          n426 = case shown="True" w918 {
            tunnel: [w920 w931] -> w917
            tunnel: w916 -> [w920 w930]
            tunnel: w915 -> [_ w928]
            tunnel: w914 -> [w919 w923]
            tunnel: [w919 w922] -> w913
            tunnel: w912 -> [_ w921]
            frame #0 {
            }
            frame #1 {
              n427 = call "E-Time.vi"() -> ("Elapsed Time (sec)"=w929:dbl)  [unwired: 9 in, 2 out]
              n428 = Subtract(x=w929, y=w928) -> (x-y=w927:dbl)
              n429 = Subtract(x=w927, y="Cooldown time") -> (x-y=w925:dbl)
              n430 = Greater Than 0?(x=w925) -> (x > 0?=w924:bool)
              n431 = case shown="True" w924 {
                tunnel: [w933 Dryer_Test_State."Wait to Start" ("Test State")] -> w931
                tunnel: w930 -> [w933 _]
                tunnel: w923 -> [w932 w938]
                tunnel: [w932 w937] -> w922
                tunnel: w921 -> [_ w934]
                frame #0 {
                }
                frame #1 {
                  n432 = call "Com Chan Type Conversion.vi"("Com Chan"=w934) -> ("VISA resource name"=w936:refnum<visa-resource-name>)  [unwired: 12 in, 2 out]
                  n433 = call "GEA2_ICP_Washer_SM.vi"("ComPort"=w936, "Mode"=GEA2_Dryer_Interface_Ctrl."Send Continue CMD", "Error In"=w938) -> ("Error Out"=w937:errorcluster)  [unwired: 7 in, 5 out]
                }
              }
            }
          }
        }
        n434 = Bundle By Name(cluster=w908, "Station Test State"=w906) -> (w907:T16)
        n435 = call <vilib>:"Clear Errors.vi"("error in (no error)"=w902) -> ("error out"=w900:errorcluster)  [unwired: 6 in]
        n436 = call <vilib>:"Add State(s) to Queue__jki_lib_state_machine.vi"("State(s) in (\"\")"=w911) -> ("States Out"=w910:string)  [unwired: 14 in]
      }
      frame #33 {
        # "If Dryer goes paused, save the test state, restore it when the dryer becomes unpaused."
        # "The check is that both string lengths are > 0. Assumes that these are initializied to \"\""
        # "Wait for both status and log to be reported."
        n437 = Unbundle By Name(w950) -> ("Station Test State"=w941:T10[], "Station Timer"=w945:dbl[], "Saved Test State"=w944:T10[])
        n438 = local read "All Test Stations"() -> (w951:T4[])
        n439 = local write "Station Test State"(w941) -> ()
        n440 = for {
          tunnel: w951 -> [w965] mode=indexing
          tunnel: [w964] -> w948 mode=indexing
          tunnel: w941 -> [w963] mode=indexing
          tunnel: [w962] -> w946 mode=indexing
          tunnel: w945 -> [w961] mode=indexing
          tunnel: w944 -> [w955] mode=indexing
          tunnel: [w954] -> w940 mode=indexing
          n441 = Unbundle By Name(w965) -> ("Dryer Details.Status"=w960:string)
          n442 = call "Type Conv - Dryer Status to Txt.vi"("Status"=Dryer_Status_Ctrl."Paused") -> ("Ring Text.Text"=w959:string)  [unwired: 10 in]
          n443 = Equal?(x=w960, y=w959) -> (x = y?=w957:bool)
          n444 = case shown="False" w957 {
            tunnel: [w967 Dryer_Test_State."Paused" ("Test State")] -> w964
            tunnel: w963 -> [w966 w973]
            tunnel: [w971 w977] -> w962
            tunnel: w961 -> [w971 _]
            tunnel: Dryer_Test_State."Paused" ("Test State") -> [w970 w976]
            tunnel: w955 -> [w968 w972]
            tunnel: [w968 w974] -> w954
            frame #0 {
              n445 = Equal?(x=w966, y=w970) -> (x = y?=w969:bool)
              n446 = Select(t=w968, s=w969, f=w966) -> (s? t:f=w967:T10)
            }
            frame #1 {
              n447 = Not Equal?(x=w973, y=w976) -> (x != y?=w975:bool)
              n448 = Select(t=w973, s=w975, f=w972) -> (s? t:f=w974:T10)
              n449 = call "E-Time.vi"() -> ("Elapsed Time (sec)"=w977:dbl)  [unwired: 9 in, 2 out]
            }
          }
        }
        n450 = Wait (ms)(milliseconds to wait=u32 500) -> ()  [unwired: 1 out]
        n451 = Bundle By Name(cluster=w950, "Station Test State"=w948, "Station Timer"=w946, "Saved Test State"=w940) -> (w949:T16)
        n452 = local write "Saved Test State"(w940) -> ()
        n453 = call <vilib>:"Add State(s) to Queue__jki_lib_state_machine.vi"("State(s) in Front (\"\")"="Start Test" ("State(s) in Front (\"\")"), "State(s) in (\"\")"=w953) -> ("States Out"=w952:string)  [unwired: 13 in]
      }
    }
    n454 = case shown="True" "Debug" {
      tunnel: w250 -> [_ w264]
      tunnel: [w261 w263] -> w249
      tunnel: w248 -> [w261 w262]
      frame #0 {
      }
      frame #1 {
        n455 = Build Array (concatenate)(w262, w264) -> (w263:string[])
        "Test State array" <- w263
      }
    }
  }
  "Test Complete" <- w3
  n456 = while "UI State Machine" {
    shift-right: [w982] -> _
    shift-left: _ -> [w981]
    shift-right: [w985] -> _
    shift-left: _ -> [w979]
    shift-right: [w984] -> _
    shift-left: w5 -> [w986]
    stop <- w983 stop-if-true
    w980 = -1  # Timeout
    n457 = call <vilib>:"Parse State Queue__jki_lib_state_machine.vi"("State Queue"=w986, "Error In (no error)"=w979) -> ("Remaining States"=w988:string, "Current State"=w989:string, "Arguments"=w987:string)  [unwired: 11 in]
    "GUI" <- w989
    n458 = case shown="\"\", \"Idle\"" w989 {
      selector: w989 -> [_ _ w1135 _ _ _]
      tunnel: w988 -> [w990 w999 w1139 w1158 w1164 w1175]
      tunnel: w987 -> [_ _ _ _ _ _]
      tunnel: w981 -> [w991 w997 w1137 w1155 w1162 _]
      tunnel: [w992 w996 w1141 errorcluster {"status"=FALSE, "code"=0, "source"=""} ("error out") w1161 w1173] -> w985
      tunnel: w979 -> [w992 w995 w1140 w1148 w1161 w1173]
      tunnel: [w990 w998 w1138 w1157 w1163 w1174] -> w984
      tunnel: [_ _ _ _ TRUE _] -> w983
      tunnel: [w991 w994 w1137 w1155 w1162 w1172] -> w982
      tunnel: w980 -> [_ w993 _ _ _ _]
      frame #0 {
        # "This state machine handles most of the the UI interrupts in the IDLE case.\n\nClicking on the dryer array elements, changes an invisible bool, which triggers the update to the name associated with\nthe dryer, or viewing the data for that dryer."
      }
      frame #1 {
        # "executes when the state queue is empty"
        n459 = event shown="[0] Timeout" {
          selector: _ -> [_ _ _ _ _ _]
          dyn-events: _ -> [_ _ _ _ _ _]
          timeout: w993 -> [_ _ _ _ _ _]
          tunnel: w999 -> [w1003 w1008 w1016 w1053 w1090 w1124]
          tunnel: [w1002 w1007 w1015 w1052 w1089 w1124] -> w998
          tunnel: w997 -> [w1000 w1005 w1013 w1050 w1087 w1125]
          tunnel: [w1001 w1006 w1014 w1051 w1088 w1120] -> w996
          tunnel: w995 -> [w1001 w1006 w1014 w1051 w1088 w1122]
          tunnel: [w1000 w1005 w1013 w1050 w1087 w1125] -> w994
          event #0 {
            n460 = event-data() -> ()  [unwired: 1 in, 1 out]
            n461 = call <vilib>:"Add State(s) to Queue__jki_lib_state_machine.vi"("State(s) in (\"\")"=w1003) -> ("States Out"=w1002:string)  [unwired: 14 in]
          }
          event #1 {
            # "Exit Button Value Change (pressed) Event\n(this executes Macro: Exit to terminate the VI)"
            n462 = event-data() -> ()  [unwired: 1 in, 1 out]
            n463 = call <vilib>:"Add State(s) to Queue__jki_lib_state_machine.vi"("State(s) in Front (\"\")"="Exit", "State(s) in (\"\")"=w1008) -> ("States Out"=w1007:string)  [unwired: 13 in]
          }
          event #2 {
            n464 = event-data() -> ()  [unwired: 1 in, 6 out]
            n465 = local read "GUI Aisle Bot"() -> (w1009:T4[])
            n466 = Array Size(array=w1009) -> (size(s)=w1012:i32)
            n467 = for {
              tunnel: w1009 -> [w1045] mode=indexing
              tunnel: [w1041] -> w1010
              i -> [w1041]
              stop <- w1042 stop-if-true
              n468 = Unbundle By Name(w1045) -> ("Boolean"=w1044:bool)
              n469 = Equal?(x=w1044, y=TRUE) -> (x = y?=w1042:bool)
            }
            n470 = Greater?(x=w1012, y=w1010) -> (0:w1011:bool)
            n471 = case shown="True" w1011 {
              tunnel: w1010 -> [_ w1022]
              tunnel: [FALSE ("FileInit") w1027] -> _
              tunnel: w1009 -> [_ w1023]
              frame #0 {
              }
              frame #1 {
                n472 = local read "Data Sample File"() -> (w1024:path)
                n473 = Index Array(array=w1023, index=w1022) -> (element=w1026:T4)
                n474 = call "Panel Washer Details.vi"("Dryer In"=w1026, "FileName"=w1024) -> ("Dryer Details Out"=w1025:T5)  [unwired: 12 in, 1 out]
                n475 = flat-sequence {
                  tunnel: w1022 -> [w1030]
                  tunnel: w1025 -> [w1031]
                  tunnel: [w1031] -> w1020
                  tunnel: [w1030] -> w1019
                  tunnel: [w1028] -> w1018
                  tunnel: [w1040] -> w1027
                  tunnel: [w1034] -> w1021
                  tunnel: w1020 -> [w1036]
                  tunnel: w1019 -> [w1035]
                  tunnel: w1018 -> [w1034]
                  frame #0 {
                    n476 = local read "2"() -> (w1029:T1)
                    n477 = call <vilib>:"Acquire Semaphore.vi"("semaphore"=w1029) -> ("semaphore out"=w1028:T1)  [unwired: 4 in, 2 out]
                  }
                  frame #1 {
                    n478 = local read "GUI Aisle Bot"() -> (w1033:T4[])
                    n479 = Index Array(array=w1033, index=w1035) -> (element=w1032:T4)
                    n480 = call "Washer HCC GUI.vi"("Washer In"=w1032, "Enum"=Update_Wilt_GUI_Control."Update Detail Data", "New Washer Details In"=w1036) -> ("Washer Out"=w1039:T4, "New Dryer Testing File Init"=w1040:bool)  [unwired: 10 in, 1 out]
                    n481 = Replace Array Subset(array=w1033, new element=w1039, index=w1035) -> (w1038:T4[])
                    n482 = local write "GUI Aisle Bot"(w1038) -> ()
                  }
                }
                n483 = call <vilib>:"Release Semaphore.vi"("semaphore"=w1021) -> ()  [unwired: 5 in, 2 out]
              }
            }
            n484 = call <vilib>:"Add State(s) to Queue__jki_lib_state_machine.vi"("State(s) in (\"\")"=w1016) -> ("States Out"=w1015:string)  [unwired: 14 in]
          }
          event #3 {
            n485 = event-data() -> ()  [unwired: 1 in, 6 out]
            n486 = local read "GUI Aisle Mid"() -> (w1046:T4[])
            n487 = Array Size(array=w1046) -> (size(s)=w1049:i32)
            n488 = for {
              tunnel: w1046 -> [w1082] mode=indexing
              tunnel: [w1078] -> w1047
              i -> [w1078]
              stop <- w1079 stop-if-true
              n489 = Unbundle By Name(w1082) -> ("Boolean"=w1081:bool)
              n490 = Equal?(x=w1081, y=TRUE) -> (x = y?=w1079:bool)
            }
            n491 = Greater?(x=w1049, y=w1047) -> (0:w1048:bool)
            n492 = case shown="True" w1048 {
              tunnel: w1047 -> [_ w1059]
              tunnel: [FALSE ("FileInit") w1064] -> _
              tunnel: w1046 -> [_ w1060]
              frame #0 {
              }
              frame #1 {
                n493 = local read "Data Sample File"() -> (w1061:path)
                n494 = Index Array(array=w1060, index=w1059) -> (element=w1063:T4)
                n495 = call "Panel Washer Details.vi"("Dryer In"=w1063, "FileName"=w1061) -> ("Dryer Details Out"=w1062:T5)  [unwired: 12 in, 1 out]
                n496 = flat-sequence {
                  tunnel: w1059 -> [w1067]
                  tunnel: w1062 -> [w1068]
                  tunnel: [w1068] -> w1057
                  tunnel: [w1067] -> w1056
                  tunnel: [w1065] -> w1055
                  tunnel: [w1077] -> w1064
                  tunnel: [w1071] -> w1058
                  tunnel: w1057 -> [w1073]
                  tunnel: w1056 -> [w1072]
                  tunnel: w1055 -> [w1071]
                  frame #0 {
                    n497 = local read "3"() -> (w1066:T1)
                    n498 = call <vilib>:"Acquire Semaphore.vi"("semaphore"=w1066) -> ("semaphore out"=w1065:T1)  [unwired: 4 in, 2 out]
                  }
                  frame #1 {
                    n499 = local read "GUI Aisle Mid"() -> (w1070:T4[])
                    n500 = Index Array(array=w1070, index=w1072) -> (element=w1069:T4)
                    n501 = call "Washer HCC GUI.vi"("Washer In"=w1069, "Enum"=Update_Wilt_GUI_Control."Update Detail Data", "New Washer Details In"=w1073) -> ("Washer Out"=w1076:T4, "New Dryer Testing File Init"=w1077:bool)  [unwired: 10 in, 1 out]
                    n502 = Replace Array Subset(array=w1070, new element=w1076, index=w1072) -> (w1075:T4[])
                    n503 = local write "GUI Aisle Mid"(w1075) -> ()
                  }
                }
                n504 = call <vilib>:"Release Semaphore.vi"("semaphore"=w1058) -> ()  [unwired: 5 in, 2 out]
              }
            }
            n505 = call <vilib>:"Add State(s) to Queue__jki_lib_state_machine.vi"("State(s) in (\"\")"=w1053) -> ("States Out"=w1052:string)  [unwired: 14 in]
          }
          event #4 {
            n506 = event-data() -> ()  [unwired: 1 in, 6 out]
            n507 = local read "GUI Aisle Top"() -> (w1083:T4[])
            n508 = Array Size(array=w1083) -> (size(s)=w1086:i32)
            n509 = for {
              tunnel: w1083 -> [w1119] mode=indexing
              tunnel: [w1115] -> w1084
              i -> [w1115]
              stop <- w1116 stop-if-true
              n510 = Unbundle By Name(w1119) -> ("Boolean"=w1118:bool)
              n511 = Equal?(x=w1118, y=TRUE) -> (x = y?=w1116:bool)
            }
            n512 = Greater?(x=w1086, y=w1084) -> (0:w1085:bool)
            n513 = case shown="True" w1085 {
              tunnel: w1084 -> [_ w1096]
              tunnel: [FALSE ("FileInit") w1101] -> _
              tunnel: w1083 -> [_ w1097]
              frame #0 {
              }
              frame #1 {
                n514 = local read "Data Sample File"() -> (w1098:path)
                n515 = Index Array(array=w1097, index=w1096) -> (element=w1100:T4)
                n516 = call "Panel Washer Details.vi"("Dryer In"=w1100, "FileName"=w1098) -> ("Dryer Details Out"=w1099:T5)  [unwired: 12 in, 1 out]
                n517 = flat-sequence {
                  tunnel: w1096 -> [w1104]
                  tunnel: w1099 -> [w1105]
                  tunnel: [w1105] -> w1094
                  tunnel: [w1104] -> w1093
                  tunnel: [w1102] -> w1092
                  tunnel: [w1114] -> w1101
                  tunnel: [w1108] -> w1095
                  tunnel: w1094 -> [w1110]
                  tunnel: w1093 -> [w1109]
                  tunnel: w1092 -> [w1108]
                  frame #0 {
                    n518 = local read "4"() -> (w1103:T1)
                    n519 = call <vilib>:"Acquire Semaphore.vi"("semaphore"=w1103) -> ("semaphore out"=w1102:T1)  [unwired: 4 in, 2 out]
                  }
                  frame #1 {
                    n520 = local read "GUI Aisle Top"() -> (w1107:T4[])
                    n521 = Index Array(array=w1107, index=w1109) -> (element=w1106:T4)
                    n522 = call "Washer HCC GUI.vi"("Washer In"=w1106, "Enum"=Update_Wilt_GUI_Control."Update Detail Data", "New Washer Details In"=w1110) -> ("Washer Out"=w1113:T4, "New Dryer Testing File Init"=w1114:bool)  [unwired: 10 in, 1 out]
                    n523 = Replace Array Subset(array=w1107, new element=w1113, index=w1109) -> (w1112:T4[])
                    n524 = local write "GUI Aisle Top"(w1112) -> ()
                  }
                }
                n525 = call <vilib>:"Release Semaphore.vi"("semaphore"=w1095) -> ()  [unwired: 5 in, 2 out]
              }
            }
            n526 = call <vilib>:"Add State(s) to Queue__jki_lib_state_machine.vi"("State(s) in (\"\")"=w1090) -> ("States Out"=w1089:string)  [unwired: 14 in]
          }
          event #5 {
            n527 = event-data() -> ()  [unwired: 1 in, 6 out]
            n528 = flat-sequence {
              tunnel: w1122 -> [w1131]
              tunnel: [w1132] -> w1121
              tunnel: [w1133] -> w1123
              tunnel: w1121 -> [w1133]
              frame #0 {
              }
              frame #1 {
                n529 = global read "Globals HCC.vi" "Path: Save File"() -> (w1127:path)
                n530 = Path To String(path=w1127) -> (string=w1130:string)
                n531 = Search and Replace String(input string="robocopy \"c:\\Data\" \"XXX\"  /S /XN" ("data backup command line"), search string="XXX", replace string=w1130) -> (result string=w1126:string)  [unwired: 5 in, 3 out]
                n532 = call <vilib>:"System Exec.vi"("error in (no error)"=w1131, "command line"=w1126) -> ("error out"=w1132:errorcluster)  [unwired: 6 in, 3 out]
              }
              frame #2 {
                n533 = local write "Robocopy"(FALSE ("Stop Test 2")) -> ()
                n534 = call <vilib>:"Simple Error Handler.vi"("error in (no error)"=w1133) -> ()  [unwired: 4 in, 5 out]
              }
            }
            n535 = call <vilib>:"Clear Errors.vi"("error in (no error)"=w1123) -> ("error out"=w1120:errorcluster)  [unwired: 6 in]
          }
        }
      }
      frame #2 {
        w1144 = 42 items=["No error", "Argument error", "Memory is full", "Out of zone", "End of file", "File already open", "Generic file I/O error", "File not found", "File permission error", "Disk is full", "Duplicate path", "Too many files open", "System feature not enabled", "Resource file not found", "Cannot add resource", "Resource not found", "Image not found", "Image memory error", "Pen does not exist", "Config type invalid", "Config token not found", "Config parse error", "Config memory error", "Bad external code format", "Bad external code offset", "External code not present", "Null window", "Destroy window error", "Null menu", "Print aborted", "Bad print record", "Print driver error", "Windows error during printing", "Memory error during printing", "Print dialog error", "Generic print error", "Invalid device refnum", "Device not found", "Device parameter error", "Device unit error", "Cannot open device", "Device call aborted", "Generic error", "Cancelled by user", "Object ID too low", "Object ID too high", "Object not in heap", "Unknown heap", "Unknown object (invalid DefProc)", "Unknown object (DefProc not in table)", "Message out of range", "Invalid (null) method", "Unknown message", "Manager call not supported", "Bad address", "Network operation in progress", "Network operation timed out", "Connection is busy", "Network attribute not supported", "Network error", "Address in use", "System out of memory", "Connection aborted", "Connection refused", "Not connected", "Already connected", "Connection closed", "Initialization error (interapplication manager)", "Bad occurrence", "Wait on unbound occurrence handler", "Occurrence queue overflow", "Datalog type conflict", "Unused", "Unrecognized type (interapplication manager)", "Memory corrupt", "Failed to make temporary DLL", "Old CIN version", "Drag socket not found", "Failed to load drop-object", "Failed to register OLE object", "Failed to release OLE object", "Format specifier type mismatch", "Unknown format specifier", "Too few format specifiers", "Too many format specifiers", "Scan failed", "Newer CIN version", "Error converting to variant", "Runtime menu error", "Password tampered", "Variant attribute not found", "Incompatible variant data type", "Event data is not available", "Event Store is not present", "Occurrence is not found", "Event Queue is not created", "Event info is not available", "Refnum passed is NULL", "Error retrieving Class GUID", "Error retrieving CoClass GUID", "Error retrieving TypeLib GUID.", "Bad built application magic bytes.", "Specific driver is different from the specific driver associated with the Logical Name.", "There is no session opened to the class driver.", "Max Error", "MAX - Error with config objects", "MAX - Error loading configuration", "MAX - Group not supported"]
        # "Current State"
        # "Do not delete, rename, or modify this frame.\n(this is used to capture unhandled states and typos)"
        # "Handle mistyped state name (developer tool)"
        n536 = Format Into String(format string="Software Exception: Unhandled State \"%s\"." ("message"), error in=w1140, w1135) -> (resulting string=w1143:string, error out=w1142:errorcluster)  [unwired: 1 in]
        n537 = call <vilib>:"Error Cluster From Error Code.vi"("show call chain? (False)"=TRUE, "error in (no error)"=w1142, "error message (\"\")"=w1143, "error code (0)"=w1144) -> ("error out"=w1141:errorcluster)  [unwired: 5 in]
        n538 = call <vilib>:"Add State(s) to Queue__jki_lib_state_machine.vi"("State(s) in (\"\")"=w1139) -> ("States Out"=w1138:string)  [unwired: 14 in]
      }
      frame #3 {
        # "Handle any errors here.\nYou can also output any states to clean-up after errors occur"
        # "Clear error"
        n539 = local read "Debug"() -> (w1146:bool)
        n540 = case shown="True" w1146 {
          tunnel: w1148 -> [_ w1159]
          frame #0 {
          }
          frame #1 {
            # "Unhandled Error -- Display it"
            n541 = call <vilib>:"General Error Handler.vi"("error in (no error)"=w1159) -> ()  [unwired: 10 in, 5 out]
          }
        }
        n542 = Unbundle By Name(w1148) -> ("source"=w1147:string)
        n543 = local read "UI Error List"() -> (w1153:string)
        n544 = Concatenate Strings("ErrorUI: " ("string"), w1147) -> (w1150:string)
        n545 = Concatenate Strings(w1147, "\n", w1153) -> (→"UI Error List":string)
        n546 = local write "User Message"(w1150) -> ()
        n547 = call <vilib>:"Add State(s) to Queue__jki_lib_state_machine.vi"("State(s) in Front (\"\")"="/* Post Error States", "State(s) in (\"\")"=w1158) -> ("States Out"=w1157:string)  [unwired: 13 in]
      }
      frame #4 {
        # "Do not put any code in this frame.\n(No errors that occur here will be handled.)"
        n548 = call <vilib>:"Add State(s) to Queue__jki_lib_state_machine.vi"("State(s) in (\"\")"=w1164) -> ("States Out"=w1163:string)  [unwired: 14 in]
      }
      frame #5 {
        n549 = flat-sequence {
          tunnel: [w1177] -> w1166
          tunnel: [w1187] -> w1171
          tunnel: [w1186] -> w1170
          tunnel: [w1185] -> w1169
          tunnel: ["Dryer To Save"] -> w1168
          tunnel: [w1188] -> w1167
          tunnel: w1166 -> [w1188]
          frame #0 {
            n550 = while {
              tunnel: [w1178] -> w1177
              stop <- w1183 stop-if-true
              n551 = local read "Gathering Data Latch"() -> (w1179:bool)
              n552 = local read "Init Complete"() -> (w1180:bool)
              n553 = local read "Test Complete"() -> (w1178:bool)
              n554 = To Unsigned Long Integer(number="DAQ Delay") -> (unsigned 32bit integer=w1182:u32)
              n555 = Wait (ms)(milliseconds to wait=w1182) -> ()  [unwired: 1 out]
              n556 = And(x=w1179, y=w1180) -> (x .and. y?=w1181:bool)
              n557 = Or(x=w1181, y=w1178) -> (x .or. y?=w1183:bool)
            }
          }
          frame #1 {
            n558 = local read "GUI Aisle Top"() -> (w1185:T4[])
            n559 = local read "GUI Aisle Mid"() -> (w1186:T4[])
            n560 = local read "GUI Aisle Bot"() -> (w1187:T4[])
          }
        }
        n561 = Bundle("GUI Aisle Bot"=w1171, "GUI Aisle Mid"=w1170, "GUI Aisle Top"=w1169, "Dryer To Save"=w1168) -> (w1172:T20)  [unwired: 1 in]
        n562 = case shown="True" w1167 {
          tunnel: [_ "Exit" ("State(s) in Front (\"\")")] -> w1165
          frame #0 {
          }
          frame #1 {
          }
        }
        n563 = call <vilib>:"Add State(s) to Queue__jki_lib_state_machine.vi"("State(s) in Front (\"\")"=w1165, "State(s) in (\"\")"=w1175) -> ("States Out"=w1174:string)  [unwired: 13 in]
      }
    }
  }
  n564 = Not(x=w3) -> (.not. x?=w4:bool)
  n565 = property on="Test Complete" class="Bool (strict)"("Val(Sgnl)"=w3) -> ()  [unwired: 2 in, 2 out]
  n566 = local write "Stop Test"(w4) -> ()
